vi "myRIO_BRig_Host_endExp_storeFiles__v5_noAnalogLabelling.vi"(0 "input_filePath":path) -> (6 "output_expPrefix":string, 8 "output_folderPath":string)   [LabVIEW 2014]
panel:
  out "error2":errorcluster
  out "error1":errorcluster
  in  "input_error":errorcluster
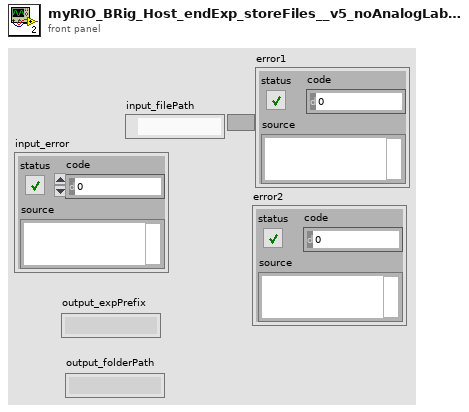
[diagram p1: front panel]
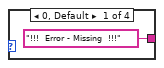
[diagram p2: hidden frame]
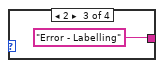
[diagram p3: hidden frame]
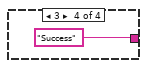
[diagram p4: hidden frame]
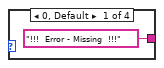
[diagram p5: hidden frame]
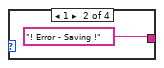
[diagram p6: hidden frame]
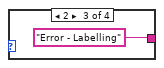
[diagram p7: hidden frame]
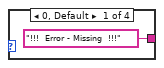
[diagram p8: hidden frame]
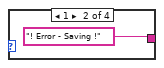
[diagram p9: hidden frame]
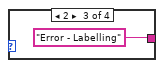
[diagram p10: hidden frame]
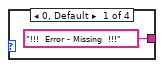
[diagram p11: hidden frame]
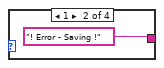
[diagram p12: hidden frame]
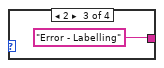
[diagram p13: hidden frame]
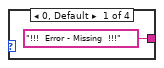
[diagram p14: hidden frame]
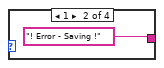
[diagram p15: hidden frame]
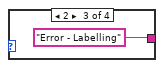
[diagram p16: hidden frame]
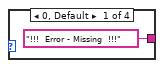
[diagram p17: hidden frame]
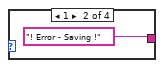
[diagram p18: hidden frame]
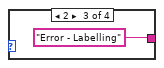
[diagram p19: hidden frame]
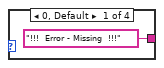
[diagram p20: hidden frame]
diagram:
  w3 = "\r"
  # "Workbooks"
  # "Application"
  # "Is Excel Running?"
  n1 = flat-sequence {
    tunnel: "input_filePath" -> [w403]
    tunnel: "input_error" -> [w401]
    tunnel: [w400] -> w395
    tunnel: [w402] -> w394
    tunnel: [w399] -> w393
    tunnel: [w398] -> w391
    tunnel: w395 -> [w446]
    tunnel: w394 -> [w447]
    tunnel: w393 -> [w407]
    tunnel: [w447] -> w392
    tunnel: w391 -> [w406]
    tunnel: [w446] -> w390
    tunnel: [w442] -> w389
    tunnel: [w441] -> w388
    tunnel: [w437] -> w314
    tunnel: [w436] -> w307
    tunnel: [w433] -> w279
    tunnel: [w430] -> w278
    tunnel: [w429] -> w277
    tunnel: [w428] -> w276
    tunnel: [w422] -> w268
    tunnel: [w421] -> w267
    tunnel: [w417] -> w266
    tunnel: [w416] -> w265
    tunnel: [w412] -> w264
    tunnel: [w411] -> w263
    tunnel: [w405] -> w40
    tunnel: [w404] -> w39
    tunnel: w392 -> [w489]
    tunnel: w390 -> [w485]
    tunnel: w389 -> [w484]
    tunnel: w388 -> [w488]
    tunnel: [w489] -> w387
    tunnel: [w487] -> w386
    tunnel: [w486] -> w385
    tunnel: [w450] -> w384
    tunnel: [w484] -> w383
    tunnel: [w483] -> w315
    tunnel: w314 -> [w483]
    tunnel: [w481] -> w308
    tunnel: w307 -> [w482]
    tunnel: [w480] -> w306
    tunnel: w279 -> [w478]
    tunnel: w278 -> [w477]
    tunnel: w277 -> [w465]
    tunnel: w276 -> [w467]
    tunnel: [w478] -> w270
    tunnel: w268 -> [w476]
    tunnel: w267 -> [w469]
    tunnel: w266 -> [w475]
    tunnel: w265 -> [w471]
    tunnel: w264 -> [w474]
    tunnel: w263 -> [w473]
    tunnel: [w464] -> w257
    tunnel: [w477] -> w251
    tunnel: [w466] -> w245
    tunnel: [w476] -> w239
    tunnel: [w468] -> w233
    tunnel: [w475] -> w227
    tunnel: [w470] -> w221
    tunnel: [w474] -> w215
    tunnel: [w472] -> w209
    tunnel: [w458] -> w208
    tunnel: [w457] -> w198
    tunnel: [w456] -> w190
    tunnel: [w455] -> w184
    tunnel: [w454] -> w179
    tunnel: [w453] -> w41
    tunnel: w40 -> [w453]
    tunnel: w39 -> [w452]
    tunnel: [w449] -> w38
    tunnel: [w448] -> w35
    tunnel: w387 -> [w531]
    tunnel: w386 -> [w529]
    tunnel: w385 -> [w528]
    tunnel: w384 -> [w495]
    tunnel: w383 -> [w530]
    tunnel: [w531] -> w370
    tunnel: [w530] -> w368
    tunnel: [w529] -> w366
    tunnel: [w528] -> w364
    tunnel: [w527] -> w362
    tunnel: [w522] -> w360
    tunnel: [w524] -> w316
    tunnel: w315 -> [w524]
    tunnel: [w525] -> w309
    tunnel: w308 -> [w525]
    tunnel: w306 -> [w526]
    tunnel: [w526] -> w305
    tunnel: [w523] -> w301
    tunnel: [w519] -> w271
    tunnel: w270 -> [w519]
    tunnel: [w520] -> w258
    tunnel: w257 -> [w520]
    tunnel: [w515] -> w252
    tunnel: w251 -> [w515]
    tunnel: [w516] -> w246
    tunnel: w245 -> [w516]
    tunnel: [w506] -> w240
    tunnel: w239 -> [w506]
    tunnel: [w509] -> w234
    tunnel: w233 -> [w509]
    tunnel: [w505] -> w228
    tunnel: w227 -> [w505]
    tunnel: [w508] -> w222
    tunnel: w221 -> [w508]
    tunnel: [w504] -> w216
    tunnel: w215 -> [w504]
    tunnel: [w507] -> w210
    tunnel: w209 -> [w507]
    tunnel: w208 -> [w521]
    tunnel: [w521] -> w204
    tunnel: [w518] -> w203
    tunnel: w198 -> [w517]
    tunnel: [w517] -> w196
    tunnel: [w514] -> w193
    tunnel: [w513] -> w191
    tunnel: w190 -> [w510]
    tunnel: [w510] -> w185
    tunnel: w184 -> [w511]
    tunnel: [w511] -> w180
    tunnel: w179 -> [w512]
    tunnel: [w512] -> w175
    tunnel: [w503] -> w174
    tunnel: [w502] -> w169
    tunnel: [w501] -> w164
    tunnel: [w500] -> w155
    tunnel: [w499] -> w153
    tunnel: [w498] -> w151
    tunnel: [w497] -> w149
    tunnel: [w496] -> w147
    tunnel: [w494] -> w42
    tunnel: w41 -> [w494]
    tunnel: w38 -> [w493]
    tunnel: [w493] -> w36
    tunnel: w35 -> [w492]
    tunnel: [w492] -> w33
    tunnel: [w491] -> w32
    tunnel: [w490] -> w31
    tunnel: w370 -> [w639]
    tunnel: [w639] -> w369
    tunnel: w368 -> [w638]
    tunnel: [w638] -> w367
    tunnel: w366 -> [w637]
    tunnel: [w637] -> w365
    tunnel: w364 -> [w636]
    tunnel: [w636] -> w363
    tunnel: w362 -> [w634]
    tunnel: [w634] -> w361
    tunnel: w360 -> [w635]
    tunnel: [w635] -> w359
    tunnel: [w630] -> w317
    tunnel: w316 -> [w630]
    tunnel: [w629] -> w310
    tunnel: w309 -> [w629]
    tunnel: w305 -> [w628]
    tunnel: [w628] -> w304
    tunnel: w301 -> [w627]
    tunnel: [w627] -> w300
    tunnel: [w626] -> w272
    tunnel: w271 -> [w626]
    tunnel: [w625] -> w259
    tunnel: w258 -> [w625]
    tunnel: [w624] -> w253
    tunnel: w252 -> [w624]
    tunnel: [w623] -> w247
    tunnel: w246 -> [w623]
    tunnel: [w622] -> w241
    tunnel: w240 -> [w622]
    tunnel: [w621] -> w235
    tunnel: w234 -> [w621]
    tunnel: [w620] -> w229
    tunnel: w228 -> [w620]
    tunnel: [w619] -> w223
    tunnel: w222 -> [w619]
    tunnel: [w618] -> w217
    tunnel: w216 -> [w618]
    tunnel: [w617] -> w211
    tunnel: w210 -> [w617]
    tunnel: [w616] -> w205
    tunnel: w204 -> [w616]
    tunnel: w203 -> [w615]
    tunnel: [w615] -> w199
    tunnel: [w614] -> w197
    tunnel: w196 -> [w614]
    tunnel: w193 -> [w606]
    tunnel: [w613] -> w192
    tunnel: w191 -> [w613]
    tunnel: [w612] -> w186
    tunnel: w185 -> [w612]
    tunnel: [w611] -> w181
    tunnel: w180 -> [w611]
    tunnel: [w610] -> w176
    tunnel: w175 -> [w610]
    tunnel: w174 -> [w609]
    tunnel: [w609] -> w170
    tunnel: w169 -> [w608]
    tunnel: [w608] -> w165
    tunnel: w164 -> [w607]
    tunnel: [w607] -> w160
    tunnel: [w606] -> w156
    tunnel: w155 -> [w605]
    tunnel: [w605] -> w154
    tunnel: w153 -> [w604]
    tunnel: [w604] -> w152
    tunnel: w151 -> [w603]
    tunnel: [w603] -> w150
    tunnel: w149 -> [w602]
    tunnel: [w602] -> w148
    tunnel: w147 -> [w601]
    tunnel: [w601] -> w146
    tunnel: [w600] -> w43
    tunnel: w42 -> [w600]
    tunnel: [w599] -> w37
    tunnel: w36 -> [w599]
    tunnel: [w598] -> w34
    tunnel: w33 -> [w598]
    tunnel: w32 -> [w596]
    tunnel: w31 -> [w597]
    tunnel: [w597] -> w30
    tunnel: [w596] -> w27
    tunnel: w369 -> [w704]
    tunnel: w367 -> [w703]
    tunnel: w365 -> [w701]
    tunnel: w363 -> [w700]
    tunnel: w361 -> [w702]
    tunnel: w359 -> [w697]
    tunnel: [w704] -> w382
    tunnel: [w703] -> w381
    tunnel: [w702] -> w380
    tunnel: [w684] -> w379
    tunnel: [w699] -> w378
    tunnel: [w698] -> w377
    tunnel: [w696] -> w318
    tunnel: w317 -> [w696]
    tunnel: [w692] -> w311
    tunnel: w310 -> [w694]
    tunnel: w304 -> [w693]
    tunnel: w300 -> [w695]
    tunnel: [w695] -> w299
    tunnel: [w691] -> w296
    tunnel: [w690] -> w273
    tunnel: w272 -> [w690]
    tunnel: [w651] -> w260
    tunnel: w259 -> [w677]
    tunnel: [w689] -> w254
    tunnel: w253 -> [w689]
    tunnel: [w654] -> w248
    tunnel: w247 -> [w674]
    tunnel: [w688] -> w242
    tunnel: w241 -> [w688]
    tunnel: [w657] -> w236
    tunnel: w235 -> [w671]
    tunnel: [w687] -> w230
    tunnel: w229 -> [w687]
    tunnel: [w660] -> w224
    tunnel: w223 -> [w668]
    tunnel: [w686] -> w218
    tunnel: w217 -> [w686]
    tunnel: [w663] -> w212
    tunnel: w211 -> [w678]
    tunnel: w205 -> [w676]
    tunnel: [w685] -> w200
    tunnel: w199 -> [w685]
    tunnel: w197 -> [w673]
    tunnel: w192 -> [w683]
    tunnel: [w662] -> w187
    tunnel: w186 -> [w665]
    tunnel: w181 -> [w667]
    tunnel: w176 -> [w670]
    tunnel: [w682] -> w171
    tunnel: w170 -> [w682]
    tunnel: [w681] -> w166
    tunnel: w165 -> [w681]
    tunnel: [w680] -> w161
    tunnel: w160 -> [w680]
    tunnel: [w679] -> w157
    tunnel: w156 -> [w679]
    tunnel: w154 -> [w675]
    tunnel: w152 -> [w672]
    tunnel: w150 -> [w669]
    tunnel: w148 -> [w666]
    tunnel: w146 -> [w664]
    tunnel: [w661] -> w145
    tunnel: [w659] -> w144
    tunnel: [w658] -> w143
    tunnel: [w656] -> w142
    tunnel: [w655] -> w141
    tunnel: [w653] -> w140
    tunnel: [w652] -> w139
    tunnel: [w650] -> w138
    tunnel: [w649] -> w137
    tunnel: [w648] -> w136
    tunnel: [w647] -> w44
    tunnel: w43 -> [w647]
    tunnel: w37 -> [w645]
    tunnel: w34 -> [w644]
    tunnel: w30 -> [w643]
    tunnel: [w646] -> w28
    tunnel: w27 -> [w646]
    tunnel: [w642] -> w24
    tunnel: [w641] -> w21
    tunnel: [w640] -> w18
    tunnel: w382 -> [w841]
    tunnel: w381 -> [w839]
    tunnel: w380 -> [w833]
    tunnel: w379 -> [w837]
    tunnel: w378 -> [w840]
    tunnel: w377 -> [w835]
    tunnel: [w841] -> w376
    tunnel: [w839] -> w375
    tunnel: [w838] -> w374
    tunnel: [w825] -> w373
    tunnel: [w840] -> w372
    tunnel: [w835] -> w371
    tunnel: [w831] -> w319
    tunnel: w318 -> [w831]
    tunnel: [w830] -> w312
    tunnel: w311 -> [w830]
    tunnel: [w826] -> w303
    tunnel: w299 -> [w828]
    tunnel: [w827] -> w298
    tunnel: w296 -> [w826]
    tunnel: [w816] -> w274
    tunnel: w273 -> [w816]
    tunnel: [w817] -> w261
    tunnel: w260 -> [w817]
    tunnel: [w809] -> w255
    tunnel: w254 -> [w809]
    tunnel: [w810] -> w249
    tunnel: w248 -> [w810]
    tunnel: [w801] -> w243
    tunnel: w242 -> [w801]
    tunnel: [w802] -> w237
    tunnel: w236 -> [w802]
    tunnel: [w788] -> w231
    tunnel: w230 -> [w788]
    tunnel: [w789] -> w225
    tunnel: w224 -> [w789]
    tunnel: [w782] -> w219
    tunnel: w218 -> [w782]
    tunnel: [w783] -> w213
    tunnel: w212 -> [w783]
    tunnel: [w819] -> w206
    tunnel: [w821] -> w201
    tunnel: w200 -> [w822]
    tunnel: [w813] -> w194
    tunnel: [w790] -> w188
    tunnel: w187 -> [w790]
    tunnel: [w791] -> w182
    tunnel: [w792] -> w177
    tunnel: [w778] -> w172
    tunnel: w171 -> [w780]
    tunnel: [w785] -> w167
    tunnel: w166 -> [w784]
    tunnel: [w798] -> w162
    tunnel: w161 -> [w799]
    tunnel: [w807] -> w158
    tunnel: w157 -> [w806]
    tunnel: w145 -> [w781]
    tunnel: w144 -> [w791]
    tunnel: w143 -> [w787]
    tunnel: w142 -> [w792]
    tunnel: w141 -> [w800]
    tunnel: w140 -> [w813]
    tunnel: w139 -> [w808]
    tunnel: w138 -> [w819]
    tunnel: w137 -> [w815]
    tunnel: w136 -> [w824]
    tunnel: [w823] -> w134
    tunnel: [w814] -> w132
    tunnel: [w805] -> w130
    tunnel: [w797] -> w128
    tunnel: [w786] -> w126
    tunnel: [w779] -> w124
    tunnel: [w771] -> w45
    tunnel: w44 -> [w771]
    tunnel: w28 -> [w773]
    tunnel: [w770] -> w25
    tunnel: w24 -> [w770]
    tunnel: [w772] -> w22
    tunnel: w21 -> [w772]
    tunnel: [w775] -> w19
    tunnel: w18 -> [w776]
    tunnel: [w774] -> w17
    tunnel: w376 -> [w941]
    tunnel: w375 -> [w946]
    tunnel: w374 -> [w945]
    tunnel: w373 -> [w944]
    tunnel: w372 -> [w943]
    tunnel: w371 -> [w942]
    tunnel: [w941] -> w358
    tunnel: [w946] -> w357
    tunnel: [w945] -> w356
    tunnel: [w944] -> w355
    tunnel: [w943] -> w354
    tunnel: [w942] -> w353
    tunnel: [w940] -> w320
    tunnel: w319 -> [w940]
    tunnel: [w939] -> w313
    tunnel: w312 -> [w939]
    tunnel: w303 -> [w938]
    tunnel: [w938] -> w302
    tunnel: w298 -> [w937]
    tunnel: [w937] -> w297
    tunnel: [w936] -> w275
    tunnel: w274 -> [w936]
    tunnel: [w935] -> w262
    tunnel: w261 -> [w935]
    tunnel: [w934] -> w256
    tunnel: w255 -> [w934]
    tunnel: [w933] -> w250
    tunnel: w249 -> [w933]
    tunnel: [w932] -> w244
    tunnel: w243 -> [w932]
    tunnel: [w931] -> w238
    tunnel: w237 -> [w931]
    tunnel: [w930] -> w232
    tunnel: w231 -> [w930]
    tunnel: [w929] -> w226
    tunnel: w225 -> [w929]
    tunnel: [w928] -> w220
    tunnel: w219 -> [w928]
    tunnel: [w927] -> w214
    tunnel: w213 -> [w927]
    tunnel: [w926] -> w207
    tunnel: w206 -> [w926]
    tunnel: [w925] -> w202
    tunnel: w201 -> [w925]
    tunnel: [w924] -> w195
    tunnel: w194 -> [w924]
    tunnel: [w923] -> w189
    tunnel: w188 -> [w923]
    tunnel: [w922] -> w183
    tunnel: w182 -> [w922]
    tunnel: [w921] -> w178
    tunnel: w177 -> [w921]
    tunnel: [w920] -> w173
    tunnel: w172 -> [w920]
    tunnel: [w919] -> w168
    tunnel: w167 -> [w919]
    tunnel: [w918] -> w163
    tunnel: w162 -> [w918]
    tunnel: [w917] -> w159
    tunnel: w158 -> [w917]
    tunnel: [w916] -> w135
    tunnel: w134 -> [w916]
    tunnel: [w915] -> w133
    tunnel: w132 -> [w915]
    tunnel: [w914] -> w131
    tunnel: w130 -> [w914]
    tunnel: [w913] -> w129
    tunnel: w128 -> [w913]
    tunnel: [w912] -> w127
    tunnel: w126 -> [w912]
    tunnel: [w911] -> w125
    tunnel: w124 -> [w911]
    tunnel: [w910] -> w46
    tunnel: w45 -> [w910]
    tunnel: [w909] -> w29
    tunnel: [w908] -> w26
    tunnel: w25 -> [w908]
    tunnel: [w907] -> w23
    tunnel: w22 -> [w907]
    tunnel: [w906] -> w20
    tunnel: w19 -> [w906]
    tunnel: w17 -> [w909]
    tunnel: w358 -> [w990]
    tunnel: w357 -> [w998]
    tunnel: w356 -> [w997]
    tunnel: w355 -> [w996]
    tunnel: w354 -> [w995]
    tunnel: w353 -> [w994]
    tunnel: [w990] -> w350
    tunnel: [w998] -> w346
    tunnel: [w997] -> w345
    tunnel: [w996] -> w342
    tunnel: [w995] -> w344
    tunnel: [w994] -> w343
    tunnel: [w986] -> w349
    tunnel: [w985] -> w348
    tunnel: [w984] -> w347
    tunnel: [w983] -> w295
    tunnel: w320 -> [w983]
    tunnel: [w982] -> w293
    tunnel: w313 -> [w982]
    tunnel: w302 -> [w981]
    tunnel: [w981] -> w292
    tunnel: w297 -> [w980]
    tunnel: [w980] -> w294
    tunnel: [w979] -> w269
    tunnel: w275 -> [w979]
    tunnel: [w978] -> w122
    tunnel: w262 -> [w978]
    tunnel: [w977] -> w120
    tunnel: w256 -> [w977]
    tunnel: [w976] -> w118
    tunnel: w250 -> [w976]
    tunnel: [w975] -> w116
    tunnel: w244 -> [w975]
    tunnel: [w974] -> w114
    tunnel: w238 -> [w974]
    tunnel: [w973] -> w112
    tunnel: w232 -> [w973]
    tunnel: [w972] -> w110
    tunnel: w226 -> [w972]
    tunnel: [w971] -> w108
    tunnel: w220 -> [w971]
    tunnel: [w970] -> w106
    tunnel: w214 -> [w970]
    tunnel: [w969] -> w121
    tunnel: w207 -> [w969]
    tunnel: [w968] -> w123
    tunnel: w202 -> [w968]
    tunnel: [w967] -> w117
    tunnel: w195 -> [w967]
    tunnel: [w966] -> w105
    tunnel: w189 -> [w966]
    tunnel: [w965] -> w109
    tunnel: w183 -> [w965]
    tunnel: [w964] -> w113
    tunnel: w178 -> [w964]
    tunnel: [w963] -> w107
    tunnel: w173 -> [w963]
    tunnel: [w962] -> w111
    tunnel: w168 -> [w962]
    tunnel: [w961] -> w115
    tunnel: w163 -> [w961]
    tunnel: [w960] -> w119
    tunnel: w159 -> [w960]
    tunnel: [w959] -> w104
    tunnel: w135 -> [w959]
    tunnel: [w958] -> w103
    tunnel: w133 -> [w958]
    tunnel: [w957] -> w102
    tunnel: w131 -> [w957]
    tunnel: [w956] -> w101
    tunnel: w129 -> [w956]
    tunnel: [w955] -> w100
    tunnel: w127 -> [w955]
    tunnel: [w954] -> w99
    tunnel: w125 -> [w954]
    tunnel: w46 -> [w953]
    tunnel: [w953] -> w16
    tunnel: [w952] -> w15
    tunnel: w29 -> [w952]
    tunnel: [w951] -> w14
    tunnel: w26 -> [w951]
    tunnel: [w950] -> w13
    tunnel: w23 -> [w950]
    tunnel: [w949] -> w12
    tunnel: w20 -> [w949]
    frame #0 {
      # "Is Excel Running?"
      # "Prepare storage"
      # "get Exp Prefix"
      n2 = call "myRIO_BRig_Host_endExp_getExp.vi"("input_filePath"=w403) -> ("output_expPrefix"=w399:string)  [unwired: 10 in]
      "output_expPrefix" <- w399
      n3 = call "myRIO_BRig_Host_isExcelRunning.vi"() -> ("output_Iexcel"=w402:bool)  [unwired: 11 in]
      n4 = call "myRIO_BRig_Host_endExp_prepareStoreLocation.vi"("input_error"=w401, "input_expPrefix"=w399) -> ("output_error"=w400:errorcluster, "output_folderPath"=w398:string)  [unwired: 8 in]
      "output_folderPath" <- w398
    }
    frame #1 {
      w408 = "dataAnalog" ("input_fileName")
      w413 = "dataTrial" ("input_fileName")
      w418 = "dataMTrig" ("input_fileName")
      w423 = "dataLick" ("input_fileName")
      w427 = "dataLC" ("input_fileName")
      w426 = "dataExp" ("input_fileName")
      w438 = "dataCurrent" ("input_fileName")
      w445 = "dataBlock" ("input_fileName")
      # "original"
      # "storage"
      # "original"
      # "storage"
      # "original"
      # "storage"
      # "original"
      # "storage"
      # "original"
      # "storage"
      # "original"
      # "storage"
      # "original"
      # "storage"
      # "original"
      # "storage"
      # "Prepare file paths"
      n5 = call "myRIO_BRig_Host_endExp_filePath__originalLocation.vi"("input_expPrefix"=w407, "input_fileName"=w426) -> ("output_filePath"=w434:string)  [unwired: 9 in]
      n6 = call "myRIO_BRig_Host_endExp_filePath__storeLocation.vi"("input_expPrefix"=w407, "input_fileName"=w426, "input_filePath_storage"=w406) -> ("output_filePath"=w435:string)  [unwired: 8 in]
      n7 = call "myRIO_BRig_Host_endExp_filePath__originalLocation.vi"("input_expPrefix"=w407, "input_fileName"=w413) -> ("output_filePath"=w414:string)  [unwired: 9 in]
      n8 = call "myRIO_BRig_Host_endExp_filePath__originalLocation.vi"("input_expPrefix"=w407, "input_fileName"=w438) -> ("output_filePath"=w439:string)  [unwired: 9 in]
      n9 = call "myRIO_BRig_Host_endExp_filePath__originalLocation.vi"("input_expPrefix"=w407, "input_fileName"=w427) -> ("output_filePath"=w431:string)  [unwired: 9 in]
      n10 = call "myRIO_BRig_Host_endExp_filePath__originalLocation.vi"("input_expPrefix"=w407, "input_fileName"=w423) -> ("output_filePath"=w424:string)  [unwired: 9 in]
      n11 = call "myRIO_BRig_Host_endExp_filePath__originalLocation.vi"("input_expPrefix"=w407, "input_fileName"=w418) -> ("output_filePath"=w419:string)  [unwired: 9 in]
      n12 = call "myRIO_BRig_Host_endExp_filePath__storeLocation.vi"("input_expPrefix"=w407, "input_fileName"=w413, "input_filePath_storage"=w406) -> ("output_filePath"=w415:string)  [unwired: 8 in]
      n13 = call "myRIO_BRig_Host_endExp_filePath__originalLocation.vi"("input_expPrefix"=w407, "input_fileName"=w408) -> ("output_filePath"=w409:string)  [unwired: 9 in]
      n14 = call "myRIO_BRig_Host_endExp_filePath__storeLocation.vi"("input_expPrefix"=w407, "input_fileName"=w438, "input_filePath_storage"=w406) -> ("output_filePath"=w440:string)  [unwired: 8 in]
      n15 = call "myRIO_BRig_Host_endExp_filePath__storeLocation.vi"("input_expPrefix"=w407, "input_fileName"=w427, "input_filePath_storage"=w406) -> ("output_filePath"=w432:string)  [unwired: 8 in]
      n16 = call "myRIO_BRig_Host_endExp_filePath__storeLocation.vi"("input_expPrefix"=w407, "input_fileName"=w423, "input_filePath_storage"=w406) -> ("output_filePath"=w425:string)  [unwired: 8 in]
      n17 = call "myRIO_BRig_Host_endExp_filePath__storeLocation.vi"("input_expPrefix"=w407, "input_fileName"=w418, "input_filePath_storage"=w406) -> ("output_filePath"=w420:string)  [unwired: 8 in]
      n18 = call "myRIO_BRig_Host_endExp_filePath__storeLocation.vi"("input_expPrefix"=w407, "input_fileName"=w408, "input_filePath_storage"=w406) -> ("output_filePath"=w410:string)  [unwired: 8 in]
      n19 = call "myRIO_BRig_Host_endExp_filePath__originalLocation.vi"("input_expPrefix"=w407, "input_fileName"=w445) -> ("output_filePath"=w443:string)  [unwired: 9 in]
      n20 = call "myRIO_BRig_Host_endExp_filePath__storeLocation.vi"("input_expPrefix"=w407, "input_fileName"=w445, "input_filePath_storage"=w406) -> ("output_filePath"=w444:string)  [unwired: 8 in]
      n21 = String To Path(string=w435) -> (path=w433:path)
      n22 = String To Path(string=w434) -> (path=w429:path)
      n23 = String To Path(string=w415) -> (path=w412:path)
      n24 = String To Path(string=w414) -> (path=w411:path)
      n25 = String To Path(string=w440) -> (path=w437:path)
      n26 = String To Path(string=w439) -> (path=w436:path)
      n27 = String To Path(string=w432) -> (path=w430:path)
      n28 = String To Path(string=w431) -> (path=w428:path)
      n29 = String To Path(string=w425) -> (path=w422:path)
      n30 = String To Path(string=w424) -> (path=w421:path)
      n31 = String To Path(string=w420) -> (path=w417:path)
      n32 = String To Path(string=w419) -> (path=w416:path)
      n33 = String To Path(string=w410) -> (path=w405:path)
      n34 = String To Path(string=w409) -> (path=w404:path)
      n35 = String To Path(string=w444) -> (path=w442:path)
      n36 = String To Path(string=w443) -> (path=w441:path)
    }
    frame #2 {
      # "Check if\noriginal files\nexist"
      n37 = call "myRIO_BRig_generic_pathExists_fast_pathInput.vi"("input_error"=w485, "input_filePath"=w488) -> ("output_error"=w479:errorcluster, "output_Iexist"=w486:bool, "output_filePath"=w487:path)  [unwired: 7 in]
      n38 = call "myRIO_BRig_generic_pathExists_fast_pathInput.vi"("input_error"=w479, "input_filePath"=w482) -> ("output_error"=w463:errorcluster, "output_Iexist"=w480:bool, "output_filePath"=w481:path)  [unwired: 7 in]
      n39 = call "myRIO_BRig_generic_pathExists_fast_pathInput.vi"("input_error"=w463, "input_filePath"=w465) -> ("output_error"=w462:errorcluster, "output_Iexist"=w458:bool, "output_filePath"=w464:path)  [unwired: 7 in]
      n40 = call "myRIO_BRig_generic_pathExists_fast_pathInput.vi"("input_error"=w462, "input_filePath"=w467) -> ("output_error"=w461:errorcluster, "output_Iexist"=w457:bool, "output_filePath"=w466:path)  [unwired: 7 in]
      n41 = call "myRIO_BRig_generic_pathExists_fast_pathInput.vi"("input_error"=w461, "input_filePath"=w469) -> ("output_error"=w460:errorcluster, "output_Iexist"=w454:bool, "output_filePath"=w468:path)  [unwired: 7 in]
      n42 = call "myRIO_BRig_generic_pathExists_fast_pathInput.vi"("input_error"=w460, "input_filePath"=w471) -> ("output_error"=w459:errorcluster, "output_Iexist"=w455:bool, "output_filePath"=w470:path)  [unwired: 7 in]
      n43 = call "myRIO_BRig_generic_pathExists_fast_pathInput.vi"("input_error"=w459, "input_filePath"=w473) -> ("output_error"=w451:errorcluster, "output_Iexist"=w456:bool, "output_filePath"=w472:path)  [unwired: 7 in]
      n44 = call "myRIO_BRig_generic_pathExists_fast_pathInput.vi"("input_error"=w451, "input_filePath"=w452) -> ("output_error"=w450:errorcluster, "output_Iexist"=w448:bool, "output_filePath"=w449:path)  [unwired: 7 in]
    }
    frame #3 {
      # "If original files exist,\nthen store them"
      n45 = case shown="True" w528 {
        selector: w528 -> [w588 w593]
        tunnel: w529 -> [_ w595]
        tunnel: w530 -> [_ w594]
        tunnel: w495 -> [w589 w592]
        tunnel: [w589 w591] -> w522
        tunnel: [w588 w590] -> w527
        frame False {
        }
        frame True {
          n46 = call "myRIO_BRig_generic_pathMove_pathInput.vi"("input_error"=w592, "input_Ioverwrite"=w593, "input_filePath_target"=w594, "input_filePath_source"=w595) -> ("output_error"=w591:errorcluster, "output_Iexist"=w590:bool)  [unwired: 5 in, 1 out]
        }
      }
      n47 = case shown="True" w526 {
        selector: w526 -> [w580 w585]
        tunnel: w525 -> [_ w587]
        tunnel: w524 -> [_ w586]
        tunnel: w495 -> [w581 w584]
        tunnel: [w581 w583] -> w513
        tunnel: [w580 w582] -> w523
        frame False {
        }
        frame True {
          n48 = call "myRIO_BRig_generic_pathMove_pathInput.vi"("input_error"=w584, "input_Ioverwrite"=w585, "input_filePath_target"=w586, "input_filePath_source"=w587) -> ("output_error"=w583:errorcluster, "output_Iexist"=w582:bool)  [unwired: 5 in, 1 out]
        }
      }
      n49 = case shown="True" w521 {
        selector: w521 -> [w572 w577]
        tunnel: w520 -> [_ w579]
        tunnel: w519 -> [_ w578]
        tunnel: w495 -> [w573 w576]
        tunnel: [w573 w575] -> w500
        tunnel: [w572 w574] -> w518
        frame False {
        }
        frame True {
          n50 = call "myRIO_BRig_generic_pathMove_pathInput.vi"("input_error"=w576, "input_Ioverwrite"=w577, "input_filePath_target"=w578, "input_filePath_source"=w579) -> ("output_error"=w575:errorcluster, "output_Iexist"=w574:bool)  [unwired: 5 in, 1 out]
        }
      }
      n51 = case shown="True" w517 {
        selector: w517 -> [w564 w569]
        tunnel: w516 -> [_ w571]
        tunnel: w515 -> [_ w570]
        tunnel: w495 -> [w565 w568]
        tunnel: [w565 w567] -> w499
        tunnel: [w564 w566] -> w514
        frame False {
        }
        frame True {
          n52 = call "myRIO_BRig_generic_pathMove_pathInput.vi"("input_error"=w568, "input_Ioverwrite"=w569, "input_filePath_target"=w570, "input_filePath_source"=w571) -> ("output_error"=w567:errorcluster, "output_Iexist"=w566:bool)  [unwired: 5 in, 1 out]
        }
      }
      n53 = case shown="True" w512 {
        selector: w512 -> [w556 w561]
        tunnel: w509 -> [_ w563]
        tunnel: w506 -> [_ w562]
        tunnel: w495 -> [w557 w560]
        tunnel: [w557 w559] -> w498
        tunnel: [w556 w558] -> w501
        frame False {
        }
        frame True {
          n54 = call "myRIO_BRig_generic_pathMove_pathInput.vi"("input_error"=w560, "input_Ioverwrite"=w561, "input_filePath_target"=w562, "input_filePath_source"=w563) -> ("output_error"=w559:errorcluster, "output_Iexist"=w558:bool)  [unwired: 5 in, 1 out]
        }
      }
      n55 = case shown="True" w511 {
        selector: w511 -> [w548 w553]
        tunnel: w508 -> [_ w555]
        tunnel: w505 -> [_ w554]
        tunnel: w495 -> [w549 w552]
        tunnel: [w549 w551] -> w497
        tunnel: [w548 w550] -> w502
        frame False {
        }
        frame True {
          n56 = call "myRIO_BRig_generic_pathMove_pathInput.vi"("input_error"=w552, "input_Ioverwrite"=w553, "input_filePath_target"=w554, "input_filePath_source"=w555) -> ("output_error"=w551:errorcluster, "output_Iexist"=w550:bool)  [unwired: 5 in, 1 out]
        }
      }
      n57 = case shown="True" w510 {
        selector: w510 -> [w540 w545]
        tunnel: w507 -> [_ w547]
        tunnel: w504 -> [_ w546]
        tunnel: w495 -> [w541 w544]
        tunnel: [w541 w543] -> w496
        tunnel: [w540 w542] -> w503
        frame False {
        }
        frame True {
          n58 = call "myRIO_BRig_generic_pathMove_pathInput.vi"("input_error"=w544, "input_Ioverwrite"=w545, "input_filePath_target"=w546, "input_filePath_source"=w547) -> ("output_error"=w543:errorcluster, "output_Iexist"=w542:bool)  [unwired: 5 in, 1 out]
        }
      }
      n59 = case shown="True" w492 {
        selector: w492 -> [w532 w537]
        tunnel: w493 -> [_ w539]
        tunnel: w494 -> [_ w538]
        tunnel: w495 -> [w533 w536]
        tunnel: [w533 w535] -> w490
        tunnel: [w532 w534] -> w491
        frame False {
        }
        frame True {
          n60 = call "myRIO_BRig_generic_pathMove_pathInput.vi"("input_error"=w536, "input_Ioverwrite"=w537, "input_filePath_target"=w538, "input_filePath_source"=w539) -> ("output_error"=w535:errorcluster, "output_Iexist"=w534:bool)  [unwired: 5 in, 1 out]
        }
      }
    }
    frame #4 {
      # "Add a delay\nin case\nall files\nweren't stored"
      n61 = Select(t=u32 0 ("milliseconds to wait"), s=w634, f=u32 200 ("milliseconds to wait")) -> (s? t:f=w633:u32)
      n62 = Wait (ms)(milliseconds to wait=w633) -> ()  [unwired: 1 out]
    }
    frame #5 {
      # "Re-check\noriginal files"
      n63 = case shown="False" w700 {
        selector: w700 -> [_ w767]
        tunnel: w701 -> [w765 w768]
        tunnel: w697 -> [w764 w766]
        tunnel: [w763 w766] -> w684
        tunnel: [w762 w768] -> w699
        tunnel: [w761 w767] -> w698
        frame False {
          n64 = call "myRIO_BRig_generic_pathExists_fast_pathInput.vi"("input_error"=w764, "input_filePath"=w765) -> ("output_error"=w763:errorcluster, "output_Iexist"=w761:bool, "output_filePath"=w762:path)  [unwired: 7 in]
        }
        frame True {
        }
      }
      n65 = case shown="False" w693 {
        selector: w693 -> [_ w759]
        tunnel: w694 -> [w757 w760]
        tunnel: w683 -> [w756 w758]
        tunnel: [w755 w758] -> w648
        tunnel: [w754 w760] -> w692
        tunnel: [w753 w759] -> w691
        frame False {
          n66 = call "myRIO_BRig_generic_pathExists_fast_pathInput.vi"("input_error"=w756, "input_filePath"=w757) -> ("output_error"=w755:errorcluster, "output_Iexist"=w753:bool, "output_filePath"=w754:path)  [unwired: 7 in]
        }
        frame True {
        }
      }
      n67 = case shown="False" w676 {
        selector: w676 -> [_ w751]
        tunnel: w677 -> [w749 w752]
        tunnel: w675 -> [w748 w750]
        tunnel: [w747 w750] -> w649
        tunnel: [w746 w752] -> w651
        tunnel: [w745 w751] -> w650
        frame False {
          n68 = call "myRIO_BRig_generic_pathExists_fast_pathInput.vi"("input_error"=w748, "input_filePath"=w749) -> ("output_error"=w747:errorcluster, "output_Iexist"=w745:bool, "output_filePath"=w746:path)  [unwired: 7 in]
        }
        frame True {
        }
      }
      n69 = case shown="False" w673 {
        selector: w673 -> [_ w743]
        tunnel: w674 -> [w741 w744]
        tunnel: w672 -> [w740 w742]
        tunnel: [w739 w742] -> w652
        tunnel: [w738 w744] -> w654
        tunnel: [w737 w743] -> w653
        frame False {
          n70 = call "myRIO_BRig_generic_pathExists_fast_pathInput.vi"("input_error"=w740, "input_filePath"=w741) -> ("output_error"=w739:errorcluster, "output_Iexist"=w737:bool, "output_filePath"=w738:path)  [unwired: 7 in]
        }
        frame True {
        }
      }
      n71 = case shown="False" w670 {
        selector: w670 -> [_ w735]
        tunnel: w671 -> [w733 w736]
        tunnel: w669 -> [w732 w734]
        tunnel: [w731 w734] -> w655
        tunnel: [w730 w736] -> w657
        tunnel: [w729 w735] -> w656
        frame False {
          n72 = call "myRIO_BRig_generic_pathExists_fast_pathInput.vi"("input_error"=w732, "input_filePath"=w733) -> ("output_error"=w731:errorcluster, "output_Iexist"=w729:bool, "output_filePath"=w730:path)  [unwired: 7 in]
        }
        frame True {
        }
      }
      n73 = case shown="False" w667 {
        selector: w667 -> [_ w727]
        tunnel: w668 -> [w725 w728]
        tunnel: w666 -> [w724 w726]
        tunnel: [w723 w726] -> w658
        tunnel: [w722 w728] -> w660
        tunnel: [w721 w727] -> w659
        frame False {
          n74 = call "myRIO_BRig_generic_pathExists_fast_pathInput.vi"("input_error"=w724, "input_filePath"=w725) -> ("output_error"=w723:errorcluster, "output_Iexist"=w721:bool, "output_filePath"=w722:path)  [unwired: 7 in]
        }
        frame True {
        }
      }
      n75 = case shown="False" w665 {
        selector: w665 -> [_ w719]
        tunnel: w678 -> [w717 w720]
        tunnel: w664 -> [w716 w718]
        tunnel: [w715 w718] -> w661
        tunnel: [w714 w720] -> w663
        tunnel: [w713 w719] -> w662
        frame False {
          n76 = call "myRIO_BRig_generic_pathExists_fast_pathInput.vi"("input_error"=w716, "input_filePath"=w717) -> ("output_error"=w715:errorcluster, "output_Iexist"=w713:bool, "output_filePath"=w714:path)  [unwired: 7 in]
        }
        frame True {
        }
      }
      n77 = case shown="False" w644 {
        selector: w644 -> [_ w711]
        tunnel: w645 -> [w709 w712]
        tunnel: w643 -> [w708 w710]
        tunnel: [w707 w710] -> w640
        tunnel: [w706 w712] -> w642
        tunnel: [w705 w711] -> w641
        frame False {
          n78 = call "myRIO_BRig_generic_pathExists_fast_pathInput.vi"("input_error"=w708, "input_filePath"=w709) -> ("output_error"=w707:errorcluster, "output_Iexist"=w705:bool, "output_filePath"=w706:path)  [unwired: 7 in]
        }
        frame True {
        }
      }
    }
    frame #6 {
      # "Re-check\nstorage"
      n79 = Not(x=w833) -> (.not. x?=w836:bool)
      n80 = Not(x=w828) -> (.not. x?=w832:bool)
      n81 = Not(x=w799) -> (.not. x?=w803:bool)
      n82 = Not(x=w784) -> (.not. x?=w796:bool)
      n83 = Not(x=w806) -> (.not. x?=w812:bool)
      n84 = Not(x=w780) -> (.not. x?=w793:bool)
      n85 = Not(x=w773) -> (.not. x?=w777:bool)
      n86 = Not(x=w822) -> (.not. x?=w820:bool)
      n87 = And(x=w836, y=w835) -> (x .and. y?=w834:bool)
      n88 = And(x=w832, y=w826) -> (x .and. y?=w829:bool)
      n89 = And(x=w803, y=w792) -> (x .and. y?=w804:bool)
      n90 = And(x=w796, y=w791) -> (x .and. y?=w795:bool)
      n91 = And(x=w812, y=w813) -> (x .and. y?=w811:bool)
      n92 = And(x=w793, y=w790) -> (x .and. y?=w794:bool)
      n93 = And(x=w777, y=w772) -> (x .and. y?=w769:bool)
      n94 = And(x=w820, y=w819) -> (x .and. y?=w818:bool)
      n95 = case shown="True" w834 {
        selector: w834 -> [_ w903]
        tunnel: w840 -> [_ w905]
        tunnel: w839 -> [_ w904]
        tunnel: w837 -> [w899 w902]
        tunnel: [w899 w901] -> w825
        tunnel: [w898 w900] -> w838
        tunnel: w833 -> [w898 _]
        frame False {
        }
        frame True {
          n96 = call "myRIO_BRig_generic_pathMove_pathInput.vi"("input_error"=w902, "input_Ioverwrite"=w903, "input_filePath_target"=w904, "input_filePath_source"=w905) -> ("output_error"=w901:errorcluster, "output_Iexist"=w900:bool)  [unwired: 5 in, 1 out]
        }
      }
      n97 = case shown="True" w829 {
        selector: w829 -> [_ w895]
        tunnel: w830 -> [_ w897]
        tunnel: w831 -> [_ w896]
        tunnel: w824 -> [w891 w894]
        tunnel: [w891 w893] -> w823
        tunnel: [w890 w892] -> w827
        tunnel: w828 -> [w890 _]
        frame False {
        }
        frame True {
          n98 = call "myRIO_BRig_generic_pathMove_pathInput.vi"("input_error"=w894, "input_Ioverwrite"=w895, "input_filePath_target"=w896, "input_filePath_source"=w897) -> ("output_error"=w893:errorcluster, "output_Iexist"=w892:bool)  [unwired: 5 in, 1 out]
        }
      }
      n99 = case shown="True" w818 {
        selector: w818 -> [_ w887]
        tunnel: w817 -> [_ w889]
        tunnel: w816 -> [_ w888]
        tunnel: w815 -> [w883 w886]
        tunnel: [w883 w885] -> w814
        tunnel: [w882 w884] -> w821
        tunnel: w822 -> [w882 _]
        frame False {
        }
        frame True {
          n100 = call "myRIO_BRig_generic_pathMove_pathInput.vi"("input_error"=w886, "input_Ioverwrite"=w887, "input_filePath_target"=w888, "input_filePath_source"=w889) -> ("output_error"=w885:errorcluster, "output_Iexist"=w884:bool)  [unwired: 5 in, 1 out]
        }
      }
      n101 = case shown="True" w811 {
        selector: w811 -> [_ w879]
        tunnel: w810 -> [_ w881]
        tunnel: w809 -> [_ w880]
        tunnel: w808 -> [w875 w878]
        tunnel: [w875 w877] -> w805
        tunnel: [w874 w876] -> w807
        tunnel: w806 -> [w874 _]
        frame False {
        }
        frame True {
          n102 = call "myRIO_BRig_generic_pathMove_pathInput.vi"("input_error"=w878, "input_Ioverwrite"=w879, "input_filePath_target"=w880, "input_filePath_source"=w881) -> ("output_error"=w877:errorcluster, "output_Iexist"=w876:bool)  [unwired: 5 in, 1 out]
        }
      }
      n103 = case shown="True" w804 {
        selector: w804 -> [_ w871]
        tunnel: w802 -> [_ w873]
        tunnel: w801 -> [_ w872]
        tunnel: w800 -> [w867 w870]
        tunnel: [w867 w869] -> w797
        tunnel: [w866 w868] -> w798
        tunnel: w799 -> [w866 _]
        frame False {
        }
        frame True {
          n104 = call "myRIO_BRig_generic_pathMove_pathInput.vi"("input_error"=w870, "input_Ioverwrite"=w871, "input_filePath_target"=w872, "input_filePath_source"=w873) -> ("output_error"=w869:errorcluster, "output_Iexist"=w868:bool)  [unwired: 5 in, 1 out]
        }
      }
      n105 = case shown="True" w795 {
        selector: w795 -> [_ w863]
        tunnel: w789 -> [_ w865]
        tunnel: w788 -> [_ w864]
        tunnel: w787 -> [w859 w862]
        tunnel: [w859 w861] -> w786
        tunnel: [w858 w860] -> w785
        tunnel: w784 -> [w858 _]
        frame False {
        }
        frame True {
          n106 = call "myRIO_BRig_generic_pathMove_pathInput.vi"("input_error"=w862, "input_Ioverwrite"=w863, "input_filePath_target"=w864, "input_filePath_source"=w865) -> ("output_error"=w861:errorcluster, "output_Iexist"=w860:bool)  [unwired: 5 in, 1 out]
        }
      }
      n107 = case shown="True" w794 {
        selector: w794 -> [_ w855]
        tunnel: w783 -> [_ w857]
        tunnel: w782 -> [_ w856]
        tunnel: w781 -> [w851 w854]
        tunnel: [w851 w853] -> w779
        tunnel: [w850 w852] -> w778
        tunnel: w780 -> [w850 _]
        frame False {
        }
        frame True {
          n108 = call "myRIO_BRig_generic_pathMove_pathInput.vi"("input_error"=w854, "input_Ioverwrite"=w855, "input_filePath_target"=w856, "input_filePath_source"=w857) -> ("output_error"=w853:errorcluster, "output_Iexist"=w852:bool)  [unwired: 5 in, 1 out]
        }
      }
      n109 = case shown="True" w769 {
        selector: w769 -> [_ w847]
        tunnel: w770 -> [_ w849]
        tunnel: w771 -> [_ w848]
        tunnel: w776 -> [w843 w846]
        tunnel: [w843 w845] -> w775
        tunnel: [w842 w844] -> w774
        tunnel: w773 -> [w842 _]
        frame False {
        }
        frame True {
          n110 = call "myRIO_BRig_generic_pathMove_pathInput.vi"("input_error"=w846, "input_Ioverwrite"=w847, "input_filePath_target"=w848, "input_filePath_source"=w849) -> ("output_error"=w845:errorcluster, "output_Iexist"=w844:bool)  [unwired: 5 in, 1 out]
        }
      }
    }
    frame #7 {
      # "Check if Excel\nis running"
      n111 = case shown="True" w941 {
        frame False {
        }
        frame True {
          n112 = One Button Dialog(message="!!! Warning !!!  Save all Excel work, then press okay\n(If Excel isn't visible, use Ctrl-Alt-Delete)", button name ("OK")="I have saved any Excel work") -> ()  [unwired: 1 out]
        }
      }
    }
    frame #8 {
      w993 = refnum<k7> refnum  # Excel._Application
      # "Is Excel Running?"
      # "Open Excel via LabView"
      # "Workbooks"
      # "Application"
      n113 = Automation Open(Automation Refnum=w993) -> (Automation Refnum=w992:refnum<k7>, error out=w991:errorcluster)  [unwired: 1 in, 2 out]
      n114 = case shown="False" w990 {
        tunnel: w992 -> [w1002 w1005]
        tunnel: w991 -> [w1001 w1004]
        tunnel: [w1000 w1004] -> w988
        tunnel: [w999 w1005] -> w987
        frame False {
          n115 = property class="_Application"(reference=w1002, error in=w1001, "Visible"=FALSE) -> (reference out=w999:refnum<k7>, error out=w1000:errorcluster)
        }
        frame True {
        }
      }
      n116 = property class="_Application"(reference=w987, error in=w988, "DisplayAlerts"=FALSE) -> (reference out=w985:refnum<k7>, error out=w986:errorcluster, "Workbooks"=w984:refnum<k7>)
    }
  }
  n117 = Unbundle By Name(w349) -> ("code"=w352:i32)
  n118 = Equal To 0?(x=w352) -> (x = 0?=w351:bool)
  n119 = case shown="True" w351 {
    tunnel: w350 -> [w1026 w1389]
    tunnel: w349 -> [w1025 w1388]
    tunnel: w348 -> [w1024 w1387]
    tunnel: w347 -> [w1023 w1386]
    tunnel: w346 -> [_ w1385]
    tunnel: w345 -> [w1021 w1384]
    tunnel: w344 -> [_ w1383]
    tunnel: w343 -> [w1020 w1382]
    tunnel: w342 -> [w1022 w1377]
    tunnel: [w1026 w1326] -> w338
    tunnel: [w1025 w1327] -> w339
    tunnel: [w1024 w1325] -> w340
    tunnel: [w1023 w1324] -> w341
    tunnel: [w1022 w1075] -> w333
    tunnel: [w1020 w1323] -> w327
    tunnel: [_ w1322] -> w328
    tunnel: [w1021 w1321] -> w329
    tunnel: w295 -> [_ w1320]
    tunnel: w294 -> [w1019 w1319]
    tunnel: w293 -> [_ w1318]
    tunnel: w292 -> [w1018 w1317]
    tunnel: [w1019 w1301] -> w285
    tunnel: [w1018 w1295] -> w283
    tunnel: [_ w1285] -> w284
    tunnel: w269 -> [_ w1283]
    tunnel: w123 -> [w1017 w1281]
    tunnel: w122 -> [_ w1279]
    tunnel: w121 -> [w1016 w1277]
    tunnel: w120 -> [_ w1275]
    tunnel: w119 -> [w1015 w1273]
    tunnel: w118 -> [_ w1271]
    tunnel: w117 -> [w1014 w1269]
    tunnel: w116 -> [_ w1267]
    tunnel: w115 -> [w1013 w1265]
    tunnel: w114 -> [_ w1263]
    tunnel: w113 -> [w1012 w1261]
    tunnel: w112 -> [_ w1259]
    tunnel: w111 -> [w1011 w1257]
    tunnel: w110 -> [_ w1255]
    tunnel: w109 -> [w1010 w1253]
    tunnel: w108 -> [_ w1251]
    tunnel: w107 -> [w1009 w1249]
    tunnel: w106 -> [_ w1247]
    tunnel: w105 -> [w1008 w1245]
    tunnel: w104 -> [_ w1244]
    tunnel: w103 -> [_ w1240]
    tunnel: w102 -> [_ w1238]
    tunnel: w101 -> [_ w1236]
    tunnel: w100 -> [_ w1234]
    tunnel: w99 -> [_ w1232]
    tunnel: [w1017 w1082] -> w52
    tunnel: [_ w1081] -> w53
    tunnel: [w1016 w1080] -> w54
    tunnel: [w1015 w1071] -> w55
    tunnel: [_ w1070] -> w56
    tunnel: [w1014 w1069] -> w57
    tunnel: [w1013 w1068] -> w58
    tunnel: [_ w1067] -> w59
    tunnel: [w1012 w1066] -> w60
    tunnel: [w1011 w1065] -> w61
    tunnel: [_ w1064] -> w62
    tunnel: [w1010 w1063] -> w63
    tunnel: [w1009 w1062] -> w66
    tunnel: [_ w1061] -> w65
    tunnel: [w1008 w1060] -> w64
    tunnel: w16 -> [_ w1059]
    tunnel: w15 -> [w1007 w1058]
    tunnel: w14 -> [_ w1057]
    tunnel: w13 -> [w1006 w1056]
    tunnel: w12 -> [_ w1055]
    tunnel: [w1007 w1028] -> w5
    tunnel: [w1006 w1027] -> w4
    frame False {
    }
    frame True {
      n120 = flat-sequence {
        tunnel: w1389 -> [w1454]
        tunnel: w1388 -> [w1451]
        tunnel: w1387 -> [w1453]
        tunnel: w1386 -> [w1445]
        tunnel: w1385 -> [w1450]
        tunnel: w1384 -> [w1449]
        tunnel: w1383 -> [w1448]
        tunnel: w1382 -> [w1447]
        tunnel: [w1454] -> w1381
        tunnel: [w1453] -> w1380
        tunnel: [w1391] -> w1379
        tunnel: [w1452] -> w1378
        tunnel: w1377 -> [w1452]
        tunnel: [w1390] -> w1376
        tunnel: [w1450] -> w1375
        tunnel: [w1449] -> w1374
        tunnel: [w1448] -> w1373
        tunnel: [w1447] -> w1372
        tunnel: [w1446] -> w1371
        tunnel: w1320 -> [w1442]
        tunnel: w1319 -> [w1441]
        tunnel: w1318 -> [w1444]
        tunnel: w1317 -> [w1443]
        tunnel: [w1442] -> w1312
        tunnel: [w1444] -> w1307
        tunnel: [w1441] -> w1306
        tunnel: [w1443] -> w1300
        tunnel: [w1440] -> w1294
        tunnel: [w1413] -> w1284
        tunnel: w1283 -> [w1413]
        tunnel: [w1412] -> w1282
        tunnel: w1281 -> [w1412]
        tunnel: [w1437] -> w1280
        tunnel: w1279 -> [w1437]
        tunnel: [w1436] -> w1278
        tunnel: w1277 -> [w1436]
        tunnel: [w1409] -> w1276
        tunnel: w1275 -> [w1409]
        tunnel: [w1408] -> w1274
        tunnel: w1273 -> [w1408]
        tunnel: [w1411] -> w1272
        tunnel: w1271 -> [w1411]
        tunnel: [w1410] -> w1270
        tunnel: w1269 -> [w1410]
        tunnel: [w1407] -> w1268
        tunnel: w1267 -> [w1407]
        tunnel: [w1406] -> w1266
        tunnel: w1265 -> [w1406]
        tunnel: [w1435] -> w1264
        tunnel: w1263 -> [w1435]
        tunnel: [w1434] -> w1262
        tunnel: w1261 -> [w1434]
        tunnel: [w1405] -> w1260
        tunnel: w1259 -> [w1405]
        tunnel: [w1404] -> w1258
        tunnel: w1257 -> [w1404]
        tunnel: [w1433] -> w1256
        tunnel: w1255 -> [w1433]
        tunnel: [w1432] -> w1254
        tunnel: w1253 -> [w1432]
        tunnel: [w1403] -> w1252
        tunnel: w1251 -> [w1403]
        tunnel: [w1402] -> w1250
        tunnel: w1249 -> [w1402]
        tunnel: [w1431] -> w1248
        tunnel: w1247 -> [w1431]
        tunnel: [w1430] -> w1246
        tunnel: w1245 -> [w1430]
        tunnel: w1244 -> [w1429]
        tunnel: [w1429] -> w1243
        tunnel: [w1428] -> w1241
        tunnel: w1240 -> [w1428]
        tunnel: [w1427] -> w1239
        tunnel: w1238 -> [w1427]
        tunnel: [w1426] -> w1237
        tunnel: w1236 -> [w1426]
        tunnel: [w1425] -> w1235
        tunnel: w1234 -> [w1425]
        tunnel: [w1424] -> w1233
        tunnel: w1232 -> [w1424]
        tunnel: [w1401] -> w1231
        tunnel: [w1400] -> w1230
        tunnel: [w1399] -> w1229
        tunnel: [w1398] -> w1228
        tunnel: [w1397] -> w1227
        tunnel: w1059 -> [w1392]
        tunnel: w1058 -> [w1393]
        tunnel: w1057 -> [w1396]
        tunnel: w1056 -> [w1395]
        tunnel: w1055 -> [w1394]
        tunnel: [w1392] -> w1050
        tunnel: [w1393] -> w1045
        tunnel: [w1396] -> w1040
        tunnel: [w1395] -> w1036
        tunnel: [w1394] -> w1031
        tunnel: w1381 -> [w1589]
        tunnel: w1380 -> [w1592]
        tunnel: w1379 -> [w1591]
        tunnel: w1378 -> [w1577]
        tunnel: w1376 -> [w1590]
        tunnel: w1375 -> [w1593]
        tunnel: w1374 -> [w1594]
        tunnel: w1373 -> [w1596]
        tunnel: w1372 -> [w1595]
        tunnel: w1371 -> [w1572]
        tunnel: [w1596] -> w1370
        tunnel: [w1595] -> w1369
        tunnel: [w1594] -> w1368
        tunnel: [w1593] -> w1367
        tunnel: [w1592] -> w1366
        tunnel: [w1591] -> w1365
        tunnel: [w1590] -> w1364
        tunnel: [w1589] -> w1363
        tunnel: [w1576] -> w1362
        tunnel: [w1574] -> w1361
        tunnel: [w1588] -> w1313
        tunnel: w1312 -> [w1588]
        tunnel: [w1587] -> w1308
        tunnel: w1307 -> [w1587]
        tunnel: w1306 -> [w1586]
        tunnel: [w1586] -> w1305
        tunnel: w1300 -> [w1585]
        tunnel: [w1585] -> w1299
        tunnel: w1294 -> [w1571]
        tunnel: [w1575] -> w1293
        tunnel: [w1573] -> w1292
        tunnel: w1284 -> [w1565]
        tunnel: w1282 -> [w1564]
        tunnel: w1280 -> [w1563]
        tunnel: w1278 -> [w1562]
        tunnel: w1276 -> [w1560]
        tunnel: w1274 -> [w1559]
        tunnel: w1272 -> [w1558]
        tunnel: w1270 -> [w1557]
        tunnel: w1268 -> [w1555]
        tunnel: w1266 -> [w1554]
        tunnel: w1264 -> [w1553]
        tunnel: w1262 -> [w1552]
        tunnel: w1260 -> [w1550]
        tunnel: w1258 -> [w1549]
        tunnel: w1256 -> [w1548]
        tunnel: w1254 -> [w1547]
        tunnel: w1252 -> [w1545]
        tunnel: w1250 -> [w1544]
        tunnel: w1248 -> [w1543]
        tunnel: w1246 -> [w1542]
        tunnel: w1243 -> [w1584]
        tunnel: [w1584] -> w1242
        tunnel: w1241 -> [w1561]
        tunnel: w1239 -> [w1556]
        tunnel: w1237 -> [w1551]
        tunnel: w1235 -> [w1546]
        tunnel: w1233 -> [w1541]
        tunnel: w1231 -> [w1570]
        tunnel: w1230 -> [w1569]
        tunnel: w1229 -> [w1568]
        tunnel: w1228 -> [w1567]
        tunnel: w1227 -> [w1566]
        tunnel: [w1525] -> w1226
        tunnel: [w1565] -> w1222
        tunnel: [w1564] -> w1218
        tunnel: [w1563] -> w1214
        tunnel: [w1562] -> w1210
        tunnel: [w1561] -> w1206
        tunnel: [w1560] -> w1202
        tunnel: [w1559] -> w1198
        tunnel: [w1558] -> w1194
        tunnel: [w1557] -> w1191
        tunnel: [w1556] -> w1187
        tunnel: [w1555] -> w1183
        tunnel: [w1554] -> w1179
        tunnel: [w1553] -> w1175
        tunnel: [w1552] -> w1171
        tunnel: [w1551] -> w1168
        tunnel: [w1550] -> w1164
        tunnel: [w1549] -> w1160
        tunnel: [w1548] -> w1156
        tunnel: [w1547] -> w1153
        tunnel: [w1546] -> w1149
        tunnel: [w1545] -> w1145
        tunnel: [w1544] -> w1141
        tunnel: [w1543] -> w1137
        tunnel: [w1542] -> w1134
        tunnel: [w1541] -> w1130
        tunnel: [w1540] -> w1122
        tunnel: [w1539] -> w1120
        tunnel: [w1538] -> w1118
        tunnel: [w1537] -> w1116
        tunnel: [w1536] -> w1114
        tunnel: [w1535] -> w1112
        tunnel: [w1534] -> w1110
        tunnel: [w1533] -> w1108
        tunnel: [w1532] -> w1106
        tunnel: [w1531] -> w1104
        tunnel: [w1530] -> w1051
        tunnel: w1050 -> [w1530]
        tunnel: [w1529] -> w1046
        tunnel: w1045 -> [w1529]
        tunnel: [w1528] -> w1041
        tunnel: w1040 -> [w1528]
        tunnel: [w1527] -> w1037
        tunnel: w1036 -> [w1527]
        tunnel: [w1526] -> w1032
        tunnel: w1031 -> [w1526]
        tunnel: w1370 -> [w1667]
        tunnel: w1369 -> [w1668]
        tunnel: w1368 -> [w1678]
        tunnel: w1367 -> [w1677]
        tunnel: w1366 -> [w1676]
        tunnel: w1365 -> [w1675]
        tunnel: w1364 -> [w1674]
        tunnel: w1363 -> [w1673]
        tunnel: w1362 -> [w1672]
        tunnel: w1361 -> [w1671]
        tunnel: [w1670] -> w1360
        tunnel: [w1669] -> w1359
        tunnel: [w1678] -> w1358
        tunnel: [w1677] -> w1357
        tunnel: [w1676] -> w1356
        tunnel: [w1675] -> w1355
        tunnel: [w1674] -> w1354
        tunnel: [w1673] -> w1353
        tunnel: [w1672] -> w1352
        tunnel: [w1671] -> w1351
        tunnel: [w1647] -> w1350
        tunnel: [w1665] -> w1314
        tunnel: w1313 -> [w1665]
        tunnel: [w1659] -> w1309
        tunnel: w1308 -> [w1661]
        tunnel: w1305 -> [w1664]
        tunnel: [w1664] -> w1304
        tunnel: w1299 -> [w1660]
        tunnel: [w1658] -> w1298
        tunnel: w1293 -> [w1663]
        tunnel: w1292 -> [w1662]
        tunnel: [w1663] -> w1289
        tunnel: [w1662] -> w1286
        tunnel: w1242 -> [w1646]
        tunnel: w1226 -> [w1666]
        tunnel: [w1657] -> w1223
        tunnel: w1222 -> [w1657]
        tunnel: [w1656] -> w1219
        tunnel: w1218 -> [w1656]
        tunnel: [w1639] -> w1215
        tunnel: w1214 -> [w1644]
        tunnel: [w1640] -> w1211
        tunnel: w1210 -> [w1643]
        tunnel: [w1641] -> w1207
        tunnel: w1206 -> [w1642]
        tunnel: [w1655] -> w1203
        tunnel: w1202 -> [w1655]
        tunnel: [w1654] -> w1199
        tunnel: w1198 -> [w1654]
        tunnel: [w1633] -> w1195
        tunnel: w1194 -> [w1638]
        tunnel: w1191 -> [w1637]
        tunnel: [w1635] -> w1188
        tunnel: w1187 -> [w1636]
        tunnel: [w1653] -> w1184
        tunnel: w1183 -> [w1653]
        tunnel: [w1652] -> w1180
        tunnel: w1179 -> [w1652]
        tunnel: [w1629] -> w1176
        tunnel: w1175 -> [w1630]
        tunnel: [w1628] -> w1172
        tunnel: w1171 -> [w1631]
        tunnel: w1168 -> [w1632]
        tunnel: [w1651] -> w1165
        tunnel: w1164 -> [w1651]
        tunnel: [w1650] -> w1161
        tunnel: w1160 -> [w1650]
        tunnel: [w1621] -> w1157
        tunnel: w1156 -> [w1626]
        tunnel: w1153 -> [w1625]
        tunnel: [w1623] -> w1150
        tunnel: w1149 -> [w1624]
        tunnel: [w1649] -> w1146
        tunnel: w1145 -> [w1649]
        tunnel: [w1648] -> w1142
        tunnel: w1141 -> [w1648]
        tunnel: [w1615] -> w1138
        tunnel: w1137 -> [w1620]
        tunnel: w1134 -> [w1619]
        tunnel: [w1617] -> w1131
        tunnel: w1130 -> [w1618]
        tunnel: [w1645] -> w1129
        tunnel: [w1634] -> w1127
        tunnel: [w1627] -> w1126
        tunnel: [w1622] -> w1125
        tunnel: [w1616] -> w1124
        tunnel: [w1614] -> w1123
        tunnel: w1122 -> [w1614]
        tunnel: [w1613] -> w1121
        tunnel: w1120 -> [w1613]
        tunnel: [w1612] -> w1119
        tunnel: w1118 -> [w1612]
        tunnel: [w1611] -> w1117
        tunnel: w1116 -> [w1611]
        tunnel: [w1610] -> w1115
        tunnel: w1114 -> [w1610]
        tunnel: [w1609] -> w1113
        tunnel: w1112 -> [w1609]
        tunnel: [w1608] -> w1111
        tunnel: w1110 -> [w1608]
        tunnel: [w1607] -> w1109
        tunnel: w1108 -> [w1607]
        tunnel: [w1606] -> w1107
        tunnel: w1106 -> [w1606]
        tunnel: [w1605] -> w1105
        tunnel: w1104 -> [w1605]
        tunnel: [w1604] -> w1052
        tunnel: w1051 -> [w1604]
        tunnel: [w1603] -> w1047
        tunnel: w1046 -> [w1603]
        tunnel: [w1599] -> w1042
        tunnel: w1041 -> [w1602]
        tunnel: w1037 -> [w1601]
        tunnel: [w1597] -> w1033
        tunnel: w1032 -> [w1600]
        tunnel: [w1598] -> w1030
        tunnel: w1360 -> [w1823]
        tunnel: w1359 -> [w1825]
        tunnel: w1358 -> [w1819]
        tunnel: w1357 -> [w1822]
        tunnel: w1356 -> [w1832]
        tunnel: w1355 -> [w1831]
        tunnel: w1354 -> [w1830]
        tunnel: w1353 -> [w1829]
        tunnel: w1352 -> [w1828]
        tunnel: w1351 -> [w1827]
        tunnel: w1350 -> [w1821]
        tunnel: [w1823] -> w1349
        tunnel: [w1825] -> w1348
        tunnel: [w1820] -> w1347
        tunnel: [w1822] -> w1346
        tunnel: [w1832] -> w1345
        tunnel: [w1831] -> w1344
        tunnel: [w1830] -> w1343
        tunnel: [w1829] -> w1342
        tunnel: [w1828] -> w1341
        tunnel: [w1827] -> w1340
        tunnel: [w1809] -> w1339
        tunnel: [w1813] -> w1315
        tunnel: w1314 -> [w1813]
        tunnel: [w1814] -> w1310
        tunnel: w1309 -> [w1814]
        tunnel: w1304 -> [w1811]
        tunnel: [w1810] -> w1303
        tunnel: w1298 -> [w1815]
        tunnel: [w1815] -> w1296
        tunnel: [w1818] -> w1290
        tunnel: w1289 -> [w1818]
        tunnel: [w1817] -> w1287
        tunnel: w1286 -> [w1817]
        tunnel: [w1775] -> w1224
        tunnel: w1223 -> [w1775]
        tunnel: [w1783] -> w1220
        tunnel: w1219 -> [w1787]
        tunnel: [w1778] -> w1216
        tunnel: w1215 -> [w1778]
        tunnel: [w1786] -> w1212
        tunnel: w1211 -> [w1786]
        tunnel: [w1779] -> w1208
        tunnel: w1207 -> [w1780]
        tunnel: [w1776] -> w1204
        tunnel: w1203 -> [w1776]
        tunnel: [w1782] -> w1200
        tunnel: w1199 -> [w1785]
        tunnel: [w1777] -> w1196
        tunnel: w1195 -> [w1777]
        tunnel: [w1784] -> w1192
        tunnel: [w1773] -> w1189
        tunnel: w1188 -> [w1774]
        tunnel: [w1759] -> w1185
        tunnel: w1184 -> [w1759]
        tunnel: [w1756] -> w1181
        tunnel: w1180 -> [w1772]
        tunnel: [w1760] -> w1177
        tunnel: w1176 -> [w1760]
        tunnel: [w1771] -> w1173
        tunnel: w1172 -> [w1771]
        tunnel: [w1757] -> w1169
        tunnel: [w1762] -> w1166
        tunnel: w1165 -> [w1762]
        tunnel: [w1754] -> w1162
        tunnel: w1161 -> [w1770]
        tunnel: [w1763] -> w1158
        tunnel: w1157 -> [w1763]
        tunnel: [w1769] -> w1154
        tunnel: [w1755] -> w1151
        tunnel: w1150 -> [w1761]
        tunnel: [w1765] -> w1147
        tunnel: w1146 -> [w1765]
        tunnel: [w1752] -> w1143
        tunnel: w1142 -> [w1768]
        tunnel: [w1766] -> w1139
        tunnel: w1138 -> [w1766]
        tunnel: [w1767] -> w1135
        tunnel: [w1753] -> w1132
        tunnel: w1131 -> [w1764]
        tunnel: w1129 -> [w1808]
        tunnel: [w1807] -> w1128
        tunnel: w1127 -> [w1784]
        tunnel: w1126 -> [w1758]
        tunnel: w1125 -> [w1769]
        tunnel: w1124 -> [w1767]
        tunnel: w1123 -> [w1798]
        tunnel: w1121 -> [w1781]
        tunnel: w1119 -> [w1799]
        tunnel: w1117 -> [w1800]
        tunnel: w1115 -> [w1801]
        tunnel: w1113 -> [w1802]
        tunnel: w1111 -> [w1803]
        tunnel: w1109 -> [w1804]
        tunnel: w1107 -> [w1805]
        tunnel: w1105 -> [w1806]
        tunnel: [w1806] -> w1102
        tunnel: [w1805] -> w1100
        tunnel: [w1804] -> w1098
        tunnel: [w1803] -> w1096
        tunnel: [w1802] -> w1094
        tunnel: [w1801] -> w1092
        tunnel: [w1800] -> w1090
        tunnel: [w1799] -> w1088
        tunnel: [w1781] -> w1086
        tunnel: [w1798] -> w1084
        tunnel: [w1743] -> w1053
        tunnel: w1052 -> [w1743]
        tunnel: [w1746] -> w1048
        tunnel: w1047 -> [w1747]
        tunnel: [w1744] -> w1043
        tunnel: w1042 -> [w1744]
        tunnel: [w1750] -> w1038
        tunnel: [w1748] -> w1034
        tunnel: w1033 -> [w1749]
        tunnel: w1030 -> [w1750]
        tunnel: w1349 -> [w1989]
        tunnel: w1348 -> [w1988]
        tunnel: w1347 -> [w1978]
        tunnel: w1346 -> [w1984]
        tunnel: w1345 -> [w1987]
        tunnel: w1344 -> [w1983]
        tunnel: w1343 -> [w1982]
        tunnel: w1342 -> [w1986]
        tunnel: w1341 -> [w1981]
        tunnel: w1340 -> [w1977]
        tunnel: w1339 -> [w1985]
        tunnel: [w1989] -> w1338
        tunnel: [w1988] -> w1337
        tunnel: [w1978] -> w1336
        tunnel: [w1984] -> w1335
        tunnel: [w1987] -> w1334
        tunnel: [w1898] -> w1333
        tunnel: [w1897] -> w1332
        tunnel: [w1986] -> w1331
        tunnel: [w1980] -> w1330
        tunnel: [w1977] -> w1329
        tunnel: [w1985] -> w1328
        tunnel: [w1969] -> w1316
        tunnel: w1315 -> [w1969]
        tunnel: [w1975] -> w1311
        tunnel: w1310 -> [w1975]
        tunnel: w1303 -> [w1971]
        tunnel: [w1971] -> w1302
        tunnel: [w1974] -> w1297
        tunnel: w1296 -> [w1974]
        tunnel: [w1965] -> w1291
        tunnel: w1290 -> [w1966]
        tunnel: [w1972] -> w1288
        tunnel: w1287 -> [w1972]
        tunnel: [w1928] -> w1225
        tunnel: w1224 -> [w1928]
        tunnel: [w1942] -> w1221
        tunnel: w1220 -> [w1942]
        tunnel: [w1964] -> w1217
        tunnel: w1216 -> [w1964]
        tunnel: [w1963] -> w1213
        tunnel: w1212 -> [w1963]
        tunnel: [w1962] -> w1209
        tunnel: w1208 -> [w1962]
        tunnel: [w1927] -> w1205
        tunnel: w1204 -> [w1927]
        tunnel: [w1939] -> w1201
        tunnel: w1200 -> [w1939]
        tunnel: [w1961] -> w1197
        tunnel: w1196 -> [w1961]
        tunnel: [w1960] -> w1193
        tunnel: w1192 -> [w1960]
        tunnel: [w1959] -> w1190
        tunnel: w1189 -> [w1959]
        tunnel: [w1923] -> w1186
        tunnel: w1185 -> [w1923]
        tunnel: [w1937] -> w1182
        tunnel: w1181 -> [w1937]
        tunnel: [w1958] -> w1178
        tunnel: w1177 -> [w1958]
        tunnel: [w1957] -> w1174
        tunnel: w1173 -> [w1957]
        tunnel: [w1956] -> w1170
        tunnel: w1169 -> [w1956]
        tunnel: [w1922] -> w1167
        tunnel: w1166 -> [w1922]
        tunnel: [w1935] -> w1163
        tunnel: w1162 -> [w1935]
        tunnel: [w1955] -> w1159
        tunnel: w1158 -> [w1955]
        tunnel: [w1954] -> w1155
        tunnel: w1154 -> [w1954]
        tunnel: [w1953] -> w1152
        tunnel: w1151 -> [w1953]
        tunnel: [w1920] -> w1148
        tunnel: w1147 -> [w1920]
        tunnel: [w1933] -> w1144
        tunnel: w1143 -> [w1933]
        tunnel: [w1952] -> w1140
        tunnel: w1139 -> [w1952]
        tunnel: [w1951] -> w1136
        tunnel: w1135 -> [w1951]
        tunnel: [w1950] -> w1133
        tunnel: w1132 -> [w1950]
        tunnel: w1128 -> [w1949]
        tunnel: [w1904] -> w1103
        tunnel: w1102 -> [w1919]
        tunnel: [w1934] -> w1101
        tunnel: w1100 -> [w1934]
        tunnel: [w1905] -> w1099
        tunnel: w1098 -> [w1921]
        tunnel: [w1936] -> w1097
        tunnel: w1096 -> [w1936]
        tunnel: [w1906] -> w1095
        tunnel: w1094 -> [w1924]
        tunnel: [w1938] -> w1093
        tunnel: w1092 -> [w1938]
        tunnel: [w1907] -> w1091
        tunnel: w1090 -> [w1925]
        tunnel: [w1940] -> w1089
        tunnel: w1088 -> [w1940]
        tunnel: [w1908] -> w1087
        tunnel: w1086 -> [w1926]
        tunnel: [w1943] -> w1085
        tunnel: w1084 -> [w1943]
        tunnel: [w1949] -> w1083
        tunnel: [w1899] -> w1054
        tunnel: w1053 -> [w1899]
        tunnel: [w1900] -> w1049
        tunnel: w1048 -> [w1900]
        tunnel: [w1903] -> w1044
        tunnel: w1043 -> [w1903]
        tunnel: [w1902] -> w1039
        tunnel: w1038 -> [w1902]
        tunnel: [w1901] -> w1035
        tunnel: w1034 -> [w1901]
        tunnel: w1338 -> [w2145]
        tunnel: w1337 -> [w2144]
        tunnel: w1336 -> [w2143]
        tunnel: w1335 -> [w2142]
        tunnel: w1334 -> [w2141]
        tunnel: w1333 -> [w2140]
        tunnel: w1332 -> [w2139]
        tunnel: w1331 -> [w2138]
        tunnel: w1330 -> [w2136]
        tunnel: w1329 -> [w2134]
        tunnel: w1328 -> [w2133]
        tunnel: [w2145] -> _
        tunnel: [w2144] -> w1323
        tunnel: [w2143] -> w1321
        tunnel: [w2142] -> _
        tunnel: [w2141] -> w1325
        tunnel: [w2140] -> w1324
        tunnel: [w2139] -> w1327
        tunnel: [w2138] -> w1326
        tunnel: [w2136] -> _
        tunnel: [w2135] -> w1322
        tunnel: [w2104] -> w1076
        tunnel: [w2132] -> _
        tunnel: w1316 -> [w2132]
        tunnel: [w2131] -> _
        tunnel: w1311 -> [w2131]
        tunnel: w1302 -> [w2130]
        tunnel: [w2130] -> w1301
        tunnel: [w2129] -> w1295
        tunnel: w1297 -> [w2129]
        tunnel: [w2126] -> _
        tunnel: w1291 -> [w2126]
        tunnel: [w2125] -> w1285
        tunnel: w1288 -> [w2127]
        tunnel: [w2124] -> _
        tunnel: w1225 -> [w2124]
        tunnel: [w2123] -> w1082
        tunnel: w1221 -> [w2123]
        tunnel: [w2122] -> _
        tunnel: w1217 -> [w2122]
        tunnel: [w2121] -> w1080
        tunnel: w1213 -> [w2121]
        tunnel: [w2080] -> w1079
        tunnel: w1209 -> [w2082]
        tunnel: [w2120] -> _
        tunnel: w1205 -> [w2120]
        tunnel: [w2119] -> w1071
        tunnel: w1201 -> [w2119]
        tunnel: [w2118] -> _
        tunnel: w1197 -> [w2118]
        tunnel: [w2117] -> w1069
        tunnel: w1193 -> [w2117]
        tunnel: [w2078] -> w1078
        tunnel: w1190 -> [w2083]
        tunnel: [w2116] -> _
        tunnel: w1186 -> [w2116]
        tunnel: [w2115] -> w1068
        tunnel: w1182 -> [w2115]
        tunnel: [w2114] -> _
        tunnel: w1178 -> [w2114]
        tunnel: [w2113] -> w1066
        tunnel: w1174 -> [w2113]
        tunnel: [w2076] -> w1074
        tunnel: w1170 -> [w2084]
        tunnel: [w2112] -> _
        tunnel: w1167 -> [w2112]
        tunnel: [w2111] -> w1065
        tunnel: w1163 -> [w2111]
        tunnel: [w2110] -> _
        tunnel: w1159 -> [w2110]
        tunnel: [w2109] -> w1063
        tunnel: w1155 -> [w2109]
        tunnel: [w2074] -> w1073
        tunnel: w1152 -> [w2085]
        tunnel: [w2108] -> _
        tunnel: w1148 -> [w2108]
        tunnel: [w2107] -> w1062
        tunnel: w1144 -> [w2107]
        tunnel: [w2106] -> _
        tunnel: w1140 -> [w2106]
        tunnel: [w2105] -> w1060
        tunnel: w1136 -> [w2105]
        tunnel: [w2072] -> w1072
        tunnel: w1133 -> [w2086]
        tunnel: [w2087] -> _
        tunnel: w1103 -> [w2087]
        tunnel: [w2073] -> w1061
        tunnel: w1101 -> [w2092]
        tunnel: [w2088] -> _
        tunnel: w1099 -> [w2088]
        tunnel: [w2075] -> w1064
        tunnel: w1097 -> [w2093]
        tunnel: [w2089] -> _
        tunnel: w1095 -> [w2089]
        tunnel: [w2077] -> w1067
        tunnel: w1093 -> [w2094]
        tunnel: [w2090] -> _
        tunnel: w1091 -> [w2090]
        tunnel: [w2079] -> w1070
        tunnel: w1089 -> [w2095]
        tunnel: [w2091] -> _
        tunnel: w1087 -> [w2091]
        tunnel: [w2081] -> w1081
        tunnel: w1085 -> [w2096]
        tunnel: w1083 -> [w2103]
        tunnel: [w2102] -> w1077
        tunnel: w1054 -> [w2071]
        tunnel: w1049 -> [w2070]
        tunnel: w1044 -> [w2069]
        tunnel: w1039 -> [w2068]
        tunnel: w1035 -> [w2067]
        tunnel: [w2071] -> _
        tunnel: [w2070] -> w1028
        tunnel: [w2069] -> _
        tunnel: [w2068] -> w1027
        tunnel: [w2067] -> w1029
        frame #0 {
          # "Use Excel\nto add\nheaders"
          n121 = case shown="True" w1449 {
            selector: w1449 -> [_ w1523]
            tunnel: w1450 -> [_ w1522]
            tunnel: w1445 -> [w1516 w1521]
            tunnel: w1451 -> [w1515 w1520]
            tunnel: [w1515 w1518] -> w1438
            tunnel: [w1516 w1519] -> w1439
            tunnel: [_ w1517] -> w1446
            frame False {
            }
            frame True {
              n122 = call "myRIO_BRig_Host_formatData_getHeaders_dataBlock.vi"() -> ("output_stringArray_dataBlock"=w1524:string[])  [unwired: 11 in]
              n123 = call "myRIO_BRig_Host_formatData_test3_p2.vi"("input_headers"=w1524, "input_error"=w1520, "input_Iexist"=w1523, "input_filePath"=w1522, "input_hdl_Workbooks"=w1521) -> ("output_error"=w1518:errorcluster, "output_newFilePath"=w1517:path, "output_hdl_Worksbooks"=w1519:refnum<k7>)  [unwired: 4 in]
            }
          }
          n124 = case shown="True" w1441 {
            selector: w1441 -> [_ w1513]
            tunnel: w1442 -> [_ w1512]
            tunnel: w1439 -> [w1506 w1511]
            tunnel: w1438 -> [w1505 w1510]
            tunnel: [w1505 w1508] -> w1422
            tunnel: [w1506 w1509] -> w1423
            tunnel: [_ w1507] -> w1440
            frame False {
            }
            frame True {
              n125 = call "myRIO_BRig_Host_formatData_getHeaders_dataCurrent.vi"() -> ("output_stringArray_dataCurrent"=w1514:string[])  [unwired: 11 in]
              n126 = call "myRIO_BRig_Host_formatData_test3_p2.vi"("input_headers"=w1514, "input_error"=w1510, "input_Iexist"=w1513, "input_filePath"=w1512, "input_hdl_Workbooks"=w1511) -> ("output_error"=w1508:errorcluster, "output_newFilePath"=w1507:path, "output_hdl_Worksbooks"=w1509:refnum<k7>)  [unwired: 4 in]
            }
          }
          n127 = case shown="True" w1412 {
            selector: w1412 -> [_ w1503]
            tunnel: w1413 -> [_ w1502]
            tunnel: w1423 -> [w1496 w1501]
            tunnel: w1422 -> [w1495 w1500]
            tunnel: [w1495 w1498] -> w1420
            tunnel: [w1496 w1499] -> w1421
            tunnel: [_ w1497] -> w1401
            frame False {
            }
            frame True {
              n128 = call "myRIO_BRig_Host_formatData_getHeaders_dataExp.vi"() -> ("output_stringArray_dataExp"=w1504:string[])  [unwired: 11 in]
              n129 = call "myRIO_BRig_Host_formatData_test3_p2.vi"("input_headers"=w1504, "input_error"=w1500, "input_Iexist"=w1503, "input_filePath"=w1502, "input_hdl_Workbooks"=w1501) -> ("output_error"=w1498:errorcluster, "output_newFilePath"=w1497:path, "output_hdl_Worksbooks"=w1499:refnum<k7>)  [unwired: 4 in]
            }
          }
          n130 = case shown="True" w1408 {
            selector: w1408 -> [_ w1493]
            tunnel: w1409 -> [_ w1492]
            tunnel: w1421 -> [w1486 w1491]
            tunnel: w1420 -> [w1485 w1490]
            tunnel: [w1485 w1488] -> w1418
            tunnel: [w1486 w1489] -> w1419
            tunnel: [_ w1487] -> w1400
            frame False {
            }
            frame True {
              n131 = call "myRIO_BRig_Host_formatData_getHeaders_dataLC.vi"() -> ("output_stringArray_dataLC"=w1494:string[])  [unwired: 11 in]
              n132 = call "myRIO_BRig_Host_formatData_test3_p2.vi"("input_headers"=w1494, "input_error"=w1490, "input_Iexist"=w1493, "input_filePath"=w1492, "input_hdl_Workbooks"=w1491) -> ("output_error"=w1488:errorcluster, "output_newFilePath"=w1487:path, "output_hdl_Worksbooks"=w1489:refnum<k7>)  [unwired: 4 in]
            }
          }
          n133 = case shown="True" w1406 {
            selector: w1406 -> [_ w1483]
            tunnel: w1407 -> [_ w1482]
            tunnel: w1419 -> [w1476 w1481]
            tunnel: w1418 -> [w1475 w1480]
            tunnel: [w1475 w1478] -> w1416
            tunnel: [w1476 w1479] -> w1417
            tunnel: [_ w1477] -> w1399
            frame False {
            }
            frame True {
              n134 = call "myRIO_BRig_Host_formatData_getHeaders_dataLick.vi"() -> ("output_stringArray_dataLick"=w1484:string[])  [unwired: 11 in]
              n135 = call "myRIO_BRig_Host_formatData_test3_p2.vi"("input_headers"=w1484, "input_error"=w1480, "input_Iexist"=w1483, "input_filePath"=w1482, "input_hdl_Workbooks"=w1481) -> ("output_error"=w1478:errorcluster, "output_newFilePath"=w1477:path, "output_hdl_Worksbooks"=w1479:refnum<k7>)  [unwired: 4 in]
            }
          }
          n136 = case shown="True" w1404 {
            selector: w1404 -> [_ w1473]
            tunnel: w1405 -> [_ w1472]
            tunnel: w1417 -> [w1466 w1471]
            tunnel: w1416 -> [w1465 w1470]
            tunnel: [w1465 w1468] -> w1414
            tunnel: [w1466 w1469] -> w1415
            tunnel: [_ w1467] -> w1398
            frame False {
            }
            frame True {
              n137 = call "myRIO_BRig_Host_formatData_getHeaders_dataMTrig.vi"() -> ("output_stringArray_dataMTrig"=w1474:string[])  [unwired: 11 in]
              n138 = call "myRIO_BRig_Host_formatData_test3_p2.vi"("input_headers"=w1474, "input_error"=w1470, "input_Iexist"=w1473, "input_filePath"=w1472, "input_hdl_Workbooks"=w1471) -> ("output_error"=w1468:errorcluster, "output_newFilePath"=w1467:path, "output_hdl_Worksbooks"=w1469:refnum<k7>)  [unwired: 4 in]
            }
          }
          n139 = case shown="True" w1402 {
            selector: w1402 -> [_ w1463]
            tunnel: w1403 -> [_ w1462]
            tunnel: w1415 -> [w1456 w1461]
            tunnel: w1414 -> [w1455 w1460]
            tunnel: [w1455 w1458] -> w1390
            tunnel: [w1456 w1459] -> w1391
            tunnel: [_ w1457] -> w1397
            frame False {
            }
            frame True {
              n140 = call "myRIO_BRig_Host_formatData_getHeaders_dataTrial.vi"() -> ("output_stringArray_dataTrial"=w1464:string[])  [unwired: 11 in]
              n141 = call "myRIO_BRig_Host_formatData_test3_p2.vi"("input_headers"=w1464, "input_error"=w1460, "input_Iexist"=w1463, "input_filePath"=w1462, "input_hdl_Workbooks"=w1461) -> ("output_error"=w1458:errorcluster, "output_newFilePath"=w1457:path, "output_hdl_Worksbooks"=w1459:refnum<k7>)  [unwired: 4 in]
            }
          }
        }
        frame #1 {
          # "Check if\nfile was\ncreated"
          n142 = call "myRIO_BRig_generic_pathExists_fast_pathInput.vi"("input_error"=w1577, "input_filePath"=w1572) -> ("output_error"=w1583:errorcluster, "output_Iexist"=w1574:bool, "output_filePath"=w1576:path)  [unwired: 7 in]
          n143 = call "myRIO_BRig_generic_pathExists_fast_pathInput.vi"("input_error"=w1583, "input_filePath"=w1571) -> ("output_error"=w1582:errorcluster, "output_Iexist"=w1573:bool, "output_filePath"=w1575:path)  [unwired: 7 in]
          n144 = call "myRIO_BRig_generic_pathExists_fast_pathInput.vi"("input_error"=w1582, "input_filePath"=w1570) -> ("output_error"=w1581:errorcluster, "output_Iexist"=w1540:bool, "output_filePath"=w1539:path)  [unwired: 7 in]
          n145 = call "myRIO_BRig_generic_pathExists_fast_pathInput.vi"("input_error"=w1581, "input_filePath"=w1569) -> ("output_error"=w1580:errorcluster, "output_Iexist"=w1538:bool, "output_filePath"=w1537:path)  [unwired: 7 in]
          n146 = call "myRIO_BRig_generic_pathExists_fast_pathInput.vi"("input_error"=w1580, "input_filePath"=w1568) -> ("output_error"=w1579:errorcluster, "output_Iexist"=w1536:bool, "output_filePath"=w1535:path)  [unwired: 7 in]
          n147 = call "myRIO_BRig_generic_pathExists_fast_pathInput.vi"("input_error"=w1579, "input_filePath"=w1567) -> ("output_error"=w1578:errorcluster, "output_Iexist"=w1534:bool, "output_filePath"=w1533:path)  [unwired: 7 in]
          n148 = call "myRIO_BRig_generic_pathExists_fast_pathInput.vi"("input_error"=w1578, "input_filePath"=w1566) -> ("output_error"=w1525:errorcluster, "output_Iexist"=w1532:bool, "output_filePath"=w1531:path)  [unwired: 7 in]
        }
        frame #2 {
          # "Re-check\noriginal files"
          n149 = case shown="False" w1601 {
            selector: w1601 -> [_ w1685]
            tunnel: w1602 -> [w1683 w1686]
            tunnel: w1600 -> [w1682 w1684]
            tunnel: [w1681 w1684] -> w1597
            tunnel: [w1680 w1686] -> w1599
            tunnel: [w1679 w1685] -> w1598
            frame False {
              n150 = call "myRIO_BRig_generic_pathExists_fast_pathInput.vi"("input_error"=w1682, "input_filePath"=w1683) -> ("output_error"=w1681:errorcluster, "output_Iexist"=w1679:bool, "output_filePath"=w1680:path)  [unwired: 7 in]
            }
            frame True {
            }
          }
          n151 = case shown="False" w1668 {
            selector: w1668 -> [_ w1741]
            tunnel: w1667 -> [w1739 w1742]
            tunnel: w1666 -> [w1738 w1740]
            tunnel: [w1737 w1740] -> w1647
            tunnel: [w1736 w1742] -> w1670
            tunnel: [w1735 w1741] -> w1669
            frame False {
              n152 = call "myRIO_BRig_generic_pathExists_fast_pathInput.vi"("input_error"=w1738, "input_filePath"=w1739) -> ("output_error"=w1737:errorcluster, "output_Iexist"=w1735:bool, "output_filePath"=w1736:path)  [unwired: 7 in]
            }
            frame True {
            }
          }
          n153 = case shown="False" w1660 {
            selector: w1660 -> [_ w1733]
            tunnel: w1661 -> [w1731 w1734]
            tunnel: w1646 -> [w1730 w1732]
            tunnel: [w1729 w1732] -> w1645
            tunnel: [w1728 w1734] -> w1659
            tunnel: [w1727 w1733] -> w1658
            frame False {
              n154 = call "myRIO_BRig_generic_pathExists_fast_pathInput.vi"("input_error"=w1730, "input_filePath"=w1731) -> ("output_error"=w1729:errorcluster, "output_Iexist"=w1727:bool, "output_filePath"=w1728:path)  [unwired: 7 in]
            }
            frame True {
            }
          }
          n155 = case shown="False" w1643 {
            selector: w1643 -> [_ w1725]
            tunnel: w1644 -> [w1723 w1726]
            tunnel: w1642 -> [w1722 w1724]
            tunnel: [w1721 w1724] -> w1641
            tunnel: [w1720 w1726] -> w1639
            tunnel: [w1719 w1725] -> w1640
            frame False {
              n156 = call "myRIO_BRig_generic_pathExists_fast_pathInput.vi"("input_error"=w1722, "input_filePath"=w1723) -> ("output_error"=w1721:errorcluster, "output_Iexist"=w1719:bool, "output_filePath"=w1720:path)  [unwired: 7 in]
            }
            frame True {
            }
          }
          n157 = case shown="False" w1637 {
            selector: w1637 -> [_ w1717]
            tunnel: w1638 -> [w1715 w1718]
            tunnel: w1636 -> [w1714 w1716]
            tunnel: [w1713 w1716] -> w1635
            tunnel: [w1712 w1718] -> w1633
            tunnel: [w1711 w1717] -> w1634
            frame False {
              n158 = call "myRIO_BRig_generic_pathExists_fast_pathInput.vi"("input_error"=w1714, "input_filePath"=w1715) -> ("output_error"=w1713:errorcluster, "output_Iexist"=w1711:bool, "output_filePath"=w1712:path)  [unwired: 7 in]
            }
            frame True {
            }
          }
          n159 = case shown="False" w1631 {
            selector: w1631 -> [_ w1709]
            tunnel: w1630 -> [w1707 w1710]
            tunnel: w1632 -> [w1706 w1708]
            tunnel: [w1705 w1708] -> w1627
            tunnel: [w1704 w1710] -> w1629
            tunnel: [w1703 w1709] -> w1628
            frame False {
              n160 = call "myRIO_BRig_generic_pathExists_fast_pathInput.vi"("input_error"=w1706, "input_filePath"=w1707) -> ("output_error"=w1705:errorcluster, "output_Iexist"=w1703:bool, "output_filePath"=w1704:path)  [unwired: 7 in]
            }
            frame True {
            }
          }
          n161 = case shown="False" w1625 {
            selector: w1625 -> [_ w1701]
            tunnel: w1626 -> [w1699 w1702]
            tunnel: w1624 -> [w1698 w1700]
            tunnel: [w1697 w1700] -> w1623
            tunnel: [w1696 w1702] -> w1621
            tunnel: [w1695 w1701] -> w1622
            frame False {
              n162 = call "myRIO_BRig_generic_pathExists_fast_pathInput.vi"("input_error"=w1698, "input_filePath"=w1699) -> ("output_error"=w1697:errorcluster, "output_Iexist"=w1695:bool, "output_filePath"=w1696:path)  [unwired: 7 in]
            }
            frame True {
            }
          }
          n163 = case shown="False" w1619 {
            selector: w1619 -> [_ w1693]
            tunnel: w1620 -> [w1691 w1694]
            tunnel: w1618 -> [w1690 w1692]
            tunnel: [w1689 w1692] -> w1617
            tunnel: [w1688 w1694] -> w1615
            tunnel: [w1687 w1693] -> w1616
            frame False {
              n164 = call "myRIO_BRig_generic_pathExists_fast_pathInput.vi"("input_error"=w1690, "input_filePath"=w1691) -> ("output_error"=w1689:errorcluster, "output_Iexist"=w1687:bool, "output_filePath"=w1688:path)  [unwired: 7 in]
            }
            frame True {
            }
          }
        }
        frame #3 {
          # "Re-check\nstorage"
          n165 = Not(x=w1819) -> (.not. x?=w1826:bool)
          n166 = Not(x=w1787) -> (.not. x?=w1797:bool)
          n167 = Not(x=w1811) -> (.not. x?=w1816:bool)
          n168 = Not(x=w1785) -> (.not. x?=w1795:bool)
          n169 = Not(x=w1772) -> (.not. x?=w1793:bool)
          n170 = Not(x=w1770) -> (.not. x?=w1791:bool)
          n171 = Not(x=w1747) -> (.not. x?=w1751:bool)
          n172 = Not(x=w1768) -> (.not. x?=w1789:bool)
          n173 = And(x=w1826, y=w1825) -> (x .and. y?=w1824:bool)
          n174 = And(x=w1797, y=w1786) -> (x .and. y?=w1796:bool)
          n175 = And(x=w1816, y=w1815) -> (x .and. y?=w1812:bool)
          n176 = And(x=w1795, y=w1784) -> (x .and. y?=w1794:bool)
          n177 = And(x=w1793, y=w1771) -> (x .and. y?=w1792:bool)
          n178 = And(x=w1791, y=w1769) -> (x .and. y?=w1790:bool)
          n179 = And(x=w1751, y=w1750) -> (x .and. y?=w1745:bool)
          n180 = And(x=w1789, y=w1767) -> (x .and. y?=w1788:bool)
          n181 = case shown="True" w1824 {
            selector: w1824 -> [_ w1894]
            tunnel: w1823 -> [_ w1896]
            tunnel: w1822 -> [_ w1895]
            tunnel: w1821 -> [w1890 w1893]
            tunnel: [w1890 w1892] -> w1809
            tunnel: [w1889 w1891] -> w1820
            tunnel: w1819 -> [w1889 _]
            frame False {
            }
            frame True {
              n182 = call "myRIO_BRig_generic_pathMove_pathInput.vi"("input_error"=w1893, "input_Ioverwrite"=w1894, "input_filePath_target"=w1895, "input_filePath_source"=w1896) -> ("output_error"=w1892:errorcluster, "output_Iexist"=w1891:bool)  [unwired: 5 in, 1 out]
            }
          }
          n183 = case shown="True" w1796 {
            selector: w1796 -> [_ w1878]
            tunnel: w1778 -> [_ w1880]
            tunnel: w1775 -> [_ w1879]
            tunnel: w1780 -> [w1874 w1877]
            tunnel: [w1874 w1876] -> w1779
            tunnel: [w1873 w1875] -> w1783
            tunnel: w1787 -> [w1873 _]
            frame False {
            }
            frame True {
              n184 = call "myRIO_BRig_generic_pathMove_pathInput.vi"("input_error"=w1877, "input_Ioverwrite"=w1878, "input_filePath_target"=w1879, "input_filePath_source"=w1880) -> ("output_error"=w1876:errorcluster, "output_Iexist"=w1875:bool)  [unwired: 5 in, 1 out]
            }
          }
          n185 = case shown="True" w1812 {
            selector: w1812 -> [_ w1886]
            tunnel: w1814 -> [_ w1888]
            tunnel: w1813 -> [_ w1887]
            tunnel: w1808 -> [w1882 w1885]
            tunnel: [w1882 w1884] -> w1807
            tunnel: [w1881 w1883] -> w1810
            tunnel: w1811 -> [w1881 _]
            frame False {
            }
            frame True {
              n186 = call "myRIO_BRig_generic_pathMove_pathInput.vi"("input_error"=w1885, "input_Ioverwrite"=w1886, "input_filePath_target"=w1887, "input_filePath_source"=w1888) -> ("output_error"=w1884:errorcluster, "output_Iexist"=w1883:bool)  [unwired: 5 in, 1 out]
            }
          }
          n187 = case shown="True" w1794 {
            selector: w1794 -> [_ w1870]
            tunnel: w1777 -> [_ w1872]
            tunnel: w1776 -> [_ w1871]
            tunnel: w1774 -> [w1866 w1869]
            tunnel: [w1866 w1868] -> w1773
            tunnel: [w1865 w1867] -> w1782
            tunnel: w1785 -> [w1865 _]
            frame False {
            }
            frame True {
              n188 = call "myRIO_BRig_generic_pathMove_pathInput.vi"("input_error"=w1869, "input_Ioverwrite"=w1870, "input_filePath_target"=w1871, "input_filePath_source"=w1872) -> ("output_error"=w1868:errorcluster, "output_Iexist"=w1867:bool)  [unwired: 5 in, 1 out]
            }
          }
          n189 = case shown="True" w1792 {
            selector: w1792 -> [_ w1862]
            tunnel: w1760 -> [_ w1864]
            tunnel: w1759 -> [_ w1863]
            tunnel: w1758 -> [w1858 w1861]
            tunnel: [w1858 w1860] -> w1757
            tunnel: [w1857 w1859] -> w1756
            tunnel: w1772 -> [w1857 _]
            frame False {
            }
            frame True {
              n190 = call "myRIO_BRig_generic_pathMove_pathInput.vi"("input_error"=w1861, "input_Ioverwrite"=w1862, "input_filePath_target"=w1863, "input_filePath_source"=w1864) -> ("output_error"=w1860:errorcluster, "output_Iexist"=w1859:bool)  [unwired: 5 in, 1 out]
            }
          }
          n191 = case shown="True" w1790 {
            selector: w1790 -> [_ w1854]
            tunnel: w1763 -> [_ w1856]
            tunnel: w1762 -> [_ w1855]
            tunnel: w1761 -> [w1850 w1853]
            tunnel: [w1850 w1852] -> w1755
            tunnel: [w1849 w1851] -> w1754
            tunnel: w1770 -> [w1849 _]
            frame False {
            }
            frame True {
              n192 = call "myRIO_BRig_generic_pathMove_pathInput.vi"("input_error"=w1853, "input_Ioverwrite"=w1854, "input_filePath_target"=w1855, "input_filePath_source"=w1856) -> ("output_error"=w1852:errorcluster, "output_Iexist"=w1851:bool)  [unwired: 5 in, 1 out]
            }
          }
          n193 = case shown="True" w1745 {
            selector: w1745 -> [_ w1838]
            tunnel: w1744 -> [_ w1840]
            tunnel: w1743 -> [_ w1839]
            tunnel: w1749 -> [w1834 w1837]
            tunnel: [w1834 w1836] -> w1748
            tunnel: [w1833 w1835] -> w1746
            tunnel: w1747 -> [w1833 _]
            frame False {
            }
            frame True {
              n194 = call "myRIO_BRig_generic_pathMove_pathInput.vi"("input_error"=w1837, "input_Ioverwrite"=w1838, "input_filePath_target"=w1839, "input_filePath_source"=w1840) -> ("output_error"=w1836:errorcluster, "output_Iexist"=w1835:bool)  [unwired: 5 in, 1 out]
            }
          }
          n195 = case shown="True" w1788 {
            selector: w1788 -> [_ w1846]
            tunnel: w1766 -> [_ w1848]
            tunnel: w1765 -> [_ w1847]
            tunnel: w1764 -> [w1842 w1845]
            tunnel: [w1842 w1844] -> w1753
            tunnel: [w1841 w1843] -> w1752
            tunnel: w1768 -> [w1841 _]
            frame False {
            }
            frame True {
              n196 = call "myRIO_BRig_generic_pathMove_pathInput.vi"("input_error"=w1845, "input_Ioverwrite"=w1846, "input_filePath_target"=w1847, "input_filePath_source"=w1848) -> ("output_error"=w1844:errorcluster, "output_Iexist"=w1843:bool)  [unwired: 5 in, 1 out]
            }
          }
        }
        frame #4 {
          # "Re-check\nlabel"
          n197 = Not(x=w1934) -> (.not. x?=w1944:bool)
          n198 = Not(x=w1936) -> (.not. x?=w1945:bool)
          n199 = And(x=w1944, y=w1933) -> (x .and. y?=w1932:bool)
          n200 = And(x=w1945, y=w1935) -> (x .and. y?=w1931:bool)
          n201 = Not(x=w1977) -> (.not. x?=w1976:bool)
          n202 = Not(x=w1938) -> (.not. x?=w1946:bool)
          n203 = Not(x=w1940) -> (.not. x?=w1947:bool)
          n204 = And(x=w1976, y=w1978) -> (x .and. y?=w1979:bool)
          n205 = Not(x=w1972) -> (.not. x?=w1973:bool)
          n206 = And(x=w1946, y=w1937) -> (x .and. y?=w1930:bool)
          n207 = Not(x=w1943) -> (.not. x?=w1948:bool)
          n208 = And(x=w1947, y=w1939) -> (x .and. y?=w1929:bool)
          n209 = And(x=w1973, y=w1971) -> (x .and. y?=w1970:bool)
          n210 = And(x=w1948, y=w1942) -> (x .and. y?=w1941:bool)
          n211 = case shown="True" w1979 {
            selector: w1979 -> [_ w2065]
            tunnel: w1984 -> [_ w2064]
            tunnel: w1983 -> [w2058 w2063]
            tunnel: w1982 -> [w2057 w2062]
            tunnel: [w2057 w2060] -> w1967
            tunnel: [w2058 w2061] -> w1968
            tunnel: [w2056 w2059] -> w1980
            tunnel: w1981 -> [w2056 _]
            frame False {
            }
            frame True {
              n212 = call "myRIO_BRig_Host_formatData_getHeaders_dataBlock.vi"() -> ("output_stringArray_dataBlock"=w2066:string[])  [unwired: 11 in]
              n213 = call "myRIO_BRig_Host_formatData_test3_p2.vi"("input_headers"=w2066, "input_error"=w2062, "input_Iexist"=w2065, "input_filePath"=w2064, "input_hdl_Workbooks"=w2063) -> ("output_error"=w2060:errorcluster, "output_newFilePath"=w2059:path, "output_hdl_Worksbooks"=w2061:refnum<k7>)  [unwired: 4 in]
            }
          }
          n214 = case shown="True" w1970 {
            selector: w1970 -> [_ w2055]
            tunnel: w1969 -> [_ w2054]
            tunnel: w1968 -> [w2047 w2053]
            tunnel: w1967 -> [w2046 w2052]
            tunnel: [w2046 w2050] -> w1918
            tunnel: [w2047 w2051] -> w1917
            tunnel: [w2045 w2049] -> w1965
            tunnel: w1966 -> [w2045 _]
            frame False {
            }
            frame True {
              n215 = call "myRIO_BRig_Host_formatData_getHeaders_dataCurrent.vi"() -> ("output_stringArray_dataCurrent"=w2048:string[])  [unwired: 11 in]
              n216 = call "myRIO_BRig_Host_formatData_test3_p2.vi"("input_headers"=w2048, "input_error"=w2052, "input_Iexist"=w2055, "input_filePath"=w2054, "input_hdl_Workbooks"=w2053) -> ("output_error"=w2050:errorcluster, "output_newFilePath"=w2049:path, "output_hdl_Worksbooks"=w2051:refnum<k7>)  [unwired: 4 in]
            }
          }
          n217 = case shown="True" w1941 {
            selector: w1941 -> [_ w2044]
            tunnel: w1928 -> [_ w2043]
            tunnel: w1917 -> [w2036 w2042]
            tunnel: w1918 -> [w2035 w2041]
            tunnel: [w2035 w2039] -> w1916
            tunnel: [w2036 w2040] -> w1915
            tunnel: [w2034 w2038] -> w1908
            tunnel: w1926 -> [w2034 _]
            frame False {
            }
            frame True {
              n218 = call "myRIO_BRig_Host_formatData_getHeaders_dataExp.vi"() -> ("output_stringArray_dataExp"=w2037:string[])  [unwired: 11 in]
              n219 = call "myRIO_BRig_Host_formatData_test3_p2.vi"("input_headers"=w2037, "input_error"=w2041, "input_Iexist"=w2044, "input_filePath"=w2043, "input_hdl_Workbooks"=w2042) -> ("output_error"=w2039:errorcluster, "output_newFilePath"=w2038:path, "output_hdl_Worksbooks"=w2040:refnum<k7>)  [unwired: 4 in]
            }
          }
          n220 = case shown="True" w1929 {
            selector: w1929 -> [_ w2033]
            tunnel: w1927 -> [_ w2032]
            tunnel: w1915 -> [w2025 w2031]
            tunnel: w1916 -> [w2024 w2030]
            tunnel: [w2024 w2028] -> w1913
            tunnel: [w2025 w2029] -> w1914
            tunnel: [w2023 w2027] -> w1907
            tunnel: w1925 -> [w2023 _]
            frame False {
            }
            frame True {
              n221 = call "myRIO_BRig_Host_formatData_getHeaders_dataLC.vi"() -> ("output_stringArray_dataLC"=w2026:string[])  [unwired: 11 in]
              n222 = call "myRIO_BRig_Host_formatData_test3_p2.vi"("input_headers"=w2026, "input_error"=w2030, "input_Iexist"=w2033, "input_filePath"=w2032, "input_hdl_Workbooks"=w2031) -> ("output_error"=w2028:errorcluster, "output_newFilePath"=w2027:path, "output_hdl_Worksbooks"=w2029:refnum<k7>)  [unwired: 4 in]
            }
          }
          n223 = case shown="True" w1930 {
            selector: w1930 -> [_ w2022]
            tunnel: w1923 -> [_ w2021]
            tunnel: w1914 -> [w2014 w2020]
            tunnel: w1913 -> [w2013 w2019]
            tunnel: [w2013 w2017] -> w1911
            tunnel: [w2014 w2018] -> w1912
            tunnel: [w2012 w2016] -> w1906
            tunnel: w1924 -> [w2012 _]
            frame False {
            }
            frame True {
              n224 = call "myRIO_BRig_Host_formatData_getHeaders_dataLick.vi"() -> ("output_stringArray_dataLick"=w2015:string[])  [unwired: 11 in]
              n225 = call "myRIO_BRig_Host_formatData_test3_p2.vi"("input_headers"=w2015, "input_error"=w2019, "input_Iexist"=w2022, "input_filePath"=w2021, "input_hdl_Workbooks"=w2020) -> ("output_error"=w2017:errorcluster, "output_newFilePath"=w2016:path, "output_hdl_Worksbooks"=w2018:refnum<k7>)  [unwired: 4 in]
            }
          }
          n226 = case shown="True" w1931 {
            selector: w1931 -> [_ w2011]
            tunnel: w1922 -> [_ w2010]
            tunnel: w1912 -> [w2003 w2009]
            tunnel: w1911 -> [w2002 w2008]
            tunnel: [w2002 w2006] -> w1909
            tunnel: [w2003 w2007] -> w1910
            tunnel: [w2001 w2005] -> w1905
            tunnel: w1921 -> [w2001 _]
            frame False {
            }
            frame True {
              n227 = call "myRIO_BRig_Host_formatData_getHeaders_dataMTrig.vi"() -> ("output_stringArray_dataMTrig"=w2004:string[])  [unwired: 11 in]
              n228 = call "myRIO_BRig_Host_formatData_test3_p2.vi"("input_headers"=w2004, "input_error"=w2008, "input_Iexist"=w2011, "input_filePath"=w2010, "input_hdl_Workbooks"=w2009) -> ("output_error"=w2006:errorcluster, "output_newFilePath"=w2005:path, "output_hdl_Worksbooks"=w2007:refnum<k7>)  [unwired: 4 in]
            }
          }
          n229 = case shown="True" w1932 {
            selector: w1932 -> [_ w2000]
            tunnel: w1920 -> [_ w1999]
            tunnel: w1910 -> [w1992 w1998]
            tunnel: w1909 -> [w1991 w1997]
            tunnel: [w1991 w1995] -> w1897
            tunnel: [w1992 w1996] -> w1898
            tunnel: [w1990 w1994] -> w1904
            tunnel: w1919 -> [w1990 _]
            frame False {
            }
            frame True {
              n230 = call "myRIO_BRig_Host_formatData_getHeaders_dataTrial.vi"() -> ("output_stringArray_dataTrial"=w1993:string[])  [unwired: 11 in]
              n231 = call "myRIO_BRig_Host_formatData_test3_p2.vi"("input_headers"=w1993, "input_error"=w1997, "input_Iexist"=w2000, "input_filePath"=w1999, "input_hdl_Workbooks"=w1998) -> ("output_error"=w1995:errorcluster, "output_newFilePath"=w1994:path, "output_hdl_Worksbooks"=w1996:refnum<k7>)  [unwired: 4 in]
            }
          }
        }
        frame #5 {
          # "Re-check\nlabel\npart2"
          n232 = Not(x=w2092) -> (.not. x?=w2097:bool)
          n233 = Not(x=w2096) -> (.not. x?=w2101:bool)
          n234 = Not(x=w2093) -> (.not. x?=w2098:bool)
          n235 = Not(x=w2095) -> (.not. x?=w2100:bool)
          n236 = Not(x=w2127) -> (.not. x?=w2128:bool)
          n237 = Not(x=w2094) -> (.not. x?=w2099:bool)
          n238 = Not(x=w2134) -> (.not. x?=w2137:bool)
          n239 = case shown="True" w2097 {
            tunnel: w2086 -> [w2146 w2151]
            tunnel: w2087 -> [_ w2150]
            tunnel: [w2146 w2149] -> w2072
            tunnel: [w2147 w2148] -> w2073
            tunnel: w2092 -> [w2147 _]
            frame False {
            }
            frame True {
              n240 = call "myRIO_BRig_generic_pathExists_fast_pathInput.vi"("input_error"=w2151, "input_filePath"=w2150) -> ("output_error"=w2149:errorcluster, "output_Iexist"=w2148:bool)  [unwired: 7 in, 1 out]
            }
          }
          n241 = case shown="True" w2101 {
            tunnel: w2082 -> [w2170 w2175]
            tunnel: w2091 -> [_ w2174]
            tunnel: [w2170 w2173] -> w2080
            tunnel: [w2171 w2172] -> w2081
            tunnel: w2096 -> [w2171 _]
            frame False {
            }
            frame True {
              n242 = call "myRIO_BRig_generic_pathExists_fast_pathInput.vi"("input_error"=w2175, "input_filePath"=w2174) -> ("output_error"=w2173:errorcluster, "output_Iexist"=w2172:bool)  [unwired: 7 in, 1 out]
            }
          }
          n243 = case shown="True" w2098 {
            tunnel: w2085 -> [w2152 w2157]
            tunnel: w2088 -> [_ w2156]
            tunnel: [w2152 w2155] -> w2074
            tunnel: [w2153 w2154] -> w2075
            tunnel: w2093 -> [w2153 _]
            frame False {
            }
            frame True {
              n244 = call "myRIO_BRig_generic_pathExists_fast_pathInput.vi"("input_error"=w2157, "input_filePath"=w2156) -> ("output_error"=w2155:errorcluster, "output_Iexist"=w2154:bool)  [unwired: 7 in, 1 out]
            }
          }
          n245 = case shown="True" w2100 {
            tunnel: w2083 -> [w2164 w2169]
            tunnel: w2090 -> [_ w2168]
            tunnel: [w2164 w2167] -> w2078
            tunnel: [w2165 w2166] -> w2079
            tunnel: w2095 -> [w2165 _]
            frame False {
            }
            frame True {
              n246 = call "myRIO_BRig_generic_pathExists_fast_pathInput.vi"("input_error"=w2169, "input_filePath"=w2168) -> ("output_error"=w2167:errorcluster, "output_Iexist"=w2166:bool)  [unwired: 7 in, 1 out]
            }
          }
          n247 = case shown="True" w2128 {
            tunnel: w2103 -> [w2176 w2181]
            tunnel: w2126 -> [_ w2180]
            tunnel: [w2176 w2179] -> w2102
            tunnel: [w2177 w2178] -> w2125
            tunnel: w2127 -> [w2177 _]
            frame False {
            }
            frame True {
              n248 = call "myRIO_BRig_generic_pathExists_fast_pathInput.vi"("input_error"=w2181, "input_filePath"=w2180) -> ("output_error"=w2179:errorcluster, "output_Iexist"=w2178:bool)  [unwired: 7 in, 1 out]
            }
          }
          n249 = case shown="True" w2099 {
            tunnel: w2084 -> [w2158 w2163]
            tunnel: w2089 -> [_ w2162]
            tunnel: [w2158 w2161] -> w2076
            tunnel: [w2159 w2160] -> w2077
            tunnel: w2094 -> [w2159 _]
            frame False {
            }
            frame True {
              n250 = call "myRIO_BRig_generic_pathExists_fast_pathInput.vi"("input_error"=w2163, "input_filePath"=w2162) -> ("output_error"=w2161:errorcluster, "output_Iexist"=w2160:bool)  [unwired: 7 in, 1 out]
            }
          }
          n251 = case shown="True" w2137 {
            tunnel: w2133 -> [w2182 w2187]
            tunnel: w2136 -> [_ w2186]
            tunnel: [w2182 w2185] -> w2104
            tunnel: [w2183 w2184] -> w2135
            tunnel: w2134 -> [w2183 _]
            frame False {
            }
            frame True {
              n252 = call "myRIO_BRig_generic_pathExists_fast_pathInput.vi"("input_error"=w2187, "input_filePath"=w2186) -> ("output_error"=w2185:errorcluster, "output_Iexist"=w2184:bool)  [unwired: 7 in, 1 out]
            }
          }
        }
      }
      n253 = Merge Errors(w1076, w1077, w1079, w1078, w1074, w1073, w1072, w1029) -> (w1075:errorcluster)
    }
  }
  "error1" <- w333
  n254 = Boolean To (0,1)(Boolean=w61) -> (0, 1=w78:i16)
  n255 = Boolean To (0,1)(Boolean=w62) -> (0, 1=w77:i16)
  n256 = Boolean To (0,1)(Boolean=w63) -> (0, 1=w76:i16)
  n257 = Boolean To (0,1)(Boolean=w329) -> (0, 1=w326:i16)
  n258 = Boolean To (0,1)(Boolean=w328) -> (0, 1=w325:i16)
  n259 = Boolean To (0,1)(Boolean=w327) -> (0, 1=w324:i16)
  n260 = Boolean To (0,1)(Boolean=w52) -> (0, 1=w96:i16)
  n261 = Boolean To (0,1)(Boolean=w53) -> (0, 1=w95:i16)
  n262 = Boolean To (0,1)(Boolean=w54) -> (0, 1=w94:i16)
  n263 = Boolean To (0,1)(Boolean=w285) -> (0, 1=w291:i16)
  n264 = Boolean To (0,1)(Boolean=w284) -> (0, 1=w290:i16)
  n265 = Boolean To (0,1)(Boolean=w283) -> (0, 1=w289:i16)
  n266 = Boolean To (0,1)(Boolean=w55) -> (0, 1=w90:i16)
  n267 = Boolean To (0,1)(Boolean=w56) -> (0, 1=w89:i16)
  n268 = Boolean To (0,1)(Boolean=w57) -> (0, 1=w88:i16)
  n269 = Boolean To (0,1)(Boolean=w58) -> (0, 1=w84:i16)
  n270 = Boolean To (0,1)(Boolean=w59) -> (0, 1=w83:i16)
  n271 = Boolean To (0,1)(Boolean=w60) -> (0, 1=w82:i16)
  n272 = Boolean To (0,1)(Boolean=w66) -> (0, 1=w72:i16)
  n273 = Boolean To (0,1)(Boolean=w65) -> (0, 1=w71:i16)
  n274 = Boolean To (0,1)(Boolean=w64) -> (0, 1=w70:i16)
  n275 = Boolean To (0,1)(Boolean=w5) -> (0, 1=w11:i16)
  n276 = Boolean To (0,1)(Boolean=FALSE) -> (0, 1=w10:i16)
  n277 = Boolean To (0,1)(Boolean=w4) -> (0, 1=w9:i16)
  n278 = Compound Arithmetic op=ADD(w78, w77, w76) -> (w75:i16)
  n279 = case shown="3" w75 {
    tunnel: ["!!!  Error - Missing  !!!" "! Error - Saving !" "Error - Labelling" "Success"] -> w74
    frame 0, Default {
    }
    frame 1 {
    }
    frame 2 {
    }
    frame 3 {
    }
  }
  n280 = Compound Arithmetic op=ADD(w326, w325, w324) -> (w323:i16)
  n281 = case shown="3" w323 {
    tunnel: ["!!!  Error - Missing  !!!" "! Error - Saving !" "Error - Labelling" "Success"] -> w322
    frame 0, Default {
    }
    frame 1 {
    }
    frame 2 {
    }
    frame 3 {
    }
  }
  n282 = Compound Arithmetic op=ADD(w96, w95, w94) -> (w93:i16)
  n283 = case shown="3" w93 {
    tunnel: ["!!!  Error - Missing  !!!" "! Error - Saving !" "Error - Labelling" "Success"] -> w92
    frame 0, Default {
    }
    frame 1 {
    }
    frame 2 {
    }
    frame 3 {
    }
  }
  n284 = Compound Arithmetic op=ADD(w291, w290, w289) -> (w288:i16)
  n285 = case shown="3" w288 {
    tunnel: ["!!!  Error - Missing  !!!" "! Error - Saving !" "Error - Labelling" "Success"] -> w287
    frame 0, Default {
    }
    frame 1 {
    }
    frame 2 {
    }
    frame 3 {
    }
  }
  n286 = Compound Arithmetic op=ADD(w90, w89, w88) -> (w87:i16)
  n287 = case shown="3" w87 {
    tunnel: ["!!!  Error - Missing  !!!" "! Error - Saving !" "Error - Labelling" "Success"] -> w86
    frame 0, Default {
    }
    frame 1 {
    }
    frame 2 {
    }
    frame 3 {
    }
  }
  n288 = Compound Arithmetic op=ADD(w84, w83, w82) -> (w81:i16)
  n289 = case shown="3" w81 {
    tunnel: ["!!!  Error - Missing  !!!" "! Error - Saving !" "Error - Labelling" "Success"] -> w80
    frame 0, Default {
    }
    frame 1 {
    }
    frame 2 {
    }
    frame 3 {
    }
  }
  n290 = Compound Arithmetic op=ADD(w72, w71, w70) -> (w69:i16)
  n291 = case shown="3" w69 {
    tunnel: ["!!!  Error - Missing  !!!" "! Error - Saving !" "Error - Labelling" "Success"] -> w68
    frame 0, Default {
    }
    frame 1 {
    }
    frame 2 {
    }
    frame 3 {
    }
  }
  n292 = Compound Arithmetic op=ADD(w11, w10, w9) -> (w8:i16)
  n293 = case shown="1" w8 {
    tunnel: ["!!!  Error - Missing  !!!" "! Error - Saving !" "Error - Labelling" "Success"] -> w7
    frame 0, Default {
    }
    frame 1 {
    }
    frame 2 {
    }
    frame 3 {
    }
  }
  n294 = case shown="False" w338 {
    tunnel: w339 -> [w2223 w2229]
    tunnel: w341 -> [w2222 w2227]
    tunnel: [w2226 w2229] -> w334
    tunnel: [w2225 w2228] -> w336
    tunnel: w340 -> [w2221 w2228]
    tunnel: [w2220 w2227] -> w337
    frame False {
      n295 = invoke class="Workbooks" method="Close"(reference=w2222, error in=w2223) -> (reference out=w2220:refnum<k7>, error out=w2224:errorcluster)  [unwired: 1 in, 1 out]
      n296 = invoke class="_Application" method="Quit"(reference=w2221, error in=w2224) -> (reference out=w2225:refnum<k7>, error out=w2226:errorcluster)  [unwired: 1 in, 1 out]
    }
    frame True {
    }
  }
  n297 = Concatenate Strings("DataMTrig = ", w74) -> (w48:string)
  n298 = Concatenate Strings("DataBlock = ", w322) -> (w282:string)
  n299 = Concatenate Strings("DataExp = ", w92) -> (w51:string)
  n300 = Concatenate Strings("DataCurrent = ", w287) -> (w281:string)
  n301 = Concatenate Strings("DataLC = ", w86) -> (w50:string)
  n302 = Concatenate Strings("DataLick = ", w80) -> (w49:string)
  n303 = Concatenate Strings("DataTrial = ", w68) -> (w47:string)
  n304 = Concatenate Strings("DataAnalog = ", w7) -> (w2:string)
  n305 = Concatenate Strings(w282, w3, w281, w3, w51, w3, w50, w3, w49, w3, w48, w3, w47, w3, w2) -> (w280:string)
  n306 = flat-sequence {
    tunnel: w280 -> [w2231]
    tunnel: [w2230] -> w98
    tunnel: w97 -> [w2230]
    frame #0 {
      n307 = One Button Dialog(message=w2231) -> ()  [unwired: 1 in, 1 out]
    }
  }
  n308 = Close Reference(reference=w337, error in (no error)=w334) -> (error out=w335:errorcluster)
  n309 = Unbundle By Name(w98) -> ("code"=w332:i32)
  n310 = Close Reference(reference=w336, error in (no error)=w335) -> (error out=w97:errorcluster)
  "error2" <- w97
  n311 = Equal?(x=w332, y=-2146827284) -> (x = y?=w330:bool)
  n312 = case shown="True" w330 {
    frame False {
    }
    frame True {
      n313 = One Button Dialog(message="Use \"Alt-Ctrl-Delete\" to close Excel") -> ()  [unwired: 1 in, 1 out]
    }
  }
